vi "Auto_calibrate.vi"(3 "Mode":T4, 5 "Traverse line":T1 {"Carrier_2 Q (l/min)" format="%#.2f"; "Row Duration (mins)" format="%#.1f"; "Row No" min=0; "Trace Gas Concentration (%)" min=0.0 format="%#_4f"; "Carrier_1 Q (l/min)" format="%#.4f"; "Start X" format="%#.2f"; "Start Y" format="%#.2f"; "Start Z" format="%#.2f"; "End X" format="%#.2f"; "End Y" format="%#.2f"; "End Z" format="%#.2f"; "Tunnel Speed" format="%#.2f"; "Averaging time (mins)" min=0.0 format="%#.2f"}) -> (0 "Error Messages":string, 1 "Status":T6, 2 "Traverse Out":T1 {"Carrier_2 Q (l/min)" format="%#.2f"; "Row Duration (mins)" format="%#.1f"; "Row No" min=0; "Trace Gas Concentration (%)" min=0.0 format="%#_4f"; "Carrier_1 Q (l/min)" format="%#.4f"; "Start X" format="%#.2f"; "Start Y" format="%#.2f"; "Start Z" format="%#.2f"; "End X" format="%#.2f"; "End Y" format="%#.2f"; "End Z" format="%#.2f"; "Tunnel Speed" format="%#.2f"; "Averaging time (mins)" min=0.0 format="%#.2f"})   [LabVIEW 2022 SP3]
uses:
  Gen Trav/Traverse_cluster.ctl
  Gen Trav/Spacing.ctl
  Controls/Multi_run_mode.ctl
  Controls/User_Specific_mode.ctl
  Controls/Auto_Calib_Type.ctl
  Gen Trav/Multi_Run_Status.ctl
  Controls/Auto_Calib_Case.ctl
  FFID/HFR500 ppm Range.ctl
  File/Setup_Filetype.ctl
  Controls/Meas input Cluster.ctl
  Controls/Inst_type.ctl
  Controls/portOrDev.ctl
  Controls/calType.ctl
  Controls/channelState.ctl
  Controls/DAQinputType.ctl
  Controls/GMU Gas Line Name.ctl
  Gen Trav/Status_Cluster.ctl
  Calibration/Calib_mode.ctl
  ADAM Client/Sub VIs/ADAM Controls/Client_Source_Status.ctl
  Controls/Setup.ctl
  Controls/Post_Process.ctl
  Controls/Save_Data.ctl
  Controls/In_Range.ctl
  Controls/App_Global.ctl
  <vilib>/Analysis/baseanly.llb/Mean (DBL).vi
  Globals/Preference_global.vi
  Globals/Extra_Commands_Global.vi
  Globals/Meas_global.vi
  Globals/Calib_global.vi
  Globals/Trav_pos_global.vi
  Globals/Dynamic_call_global.ph.vi
  <vilib>/Analysis/NI_AALBase.lvlib
  <vilib>/Analysis/NI_AALPro.lvlib
panel:
  in  "stop":bool
  in  "Tab Control":enum32{"Page 1", "Page 2", "FFID"}(tab)
  out "Calibration varying":T5
  out "No of Calib Points":i32
  out "Currently On":i32
  out "Currently in Case":T7
  in  "Clear Calib History":bool
  out "New Calib Filenames":path[](array[path])
  out "Root Name":string[](array[string])
  out "Ch No's":string[](array[string])
  out "Wait factor":dbl
  out "Orig Calib file string":string
  out "Coefficients":dbl[][](array[numeric]) format="%.2f"
  out "Concentrations":dbl[](array[numeric])
  out "ppm/%Density":dbl[](array[numeric])
  out "FF Indexes":i16[](array[numeric])
  out "Values":dbl[][](array[numeric]) format="%.2f"
  out "FFID St Dev":dbl[][](array[numeric]) format="%.2f"
  out "Minimum St Dev":dbl[](array[numeric])
  out "Trace Gas %":dbl
  out "HFR500 Comms Channels":i32[](array[numeric])
  out "Multi FFID Range":bool
  in  "High Range ppm":T8=enum."5,000"
  in  "Slope less than":dbl=0.03
  in  "St Dev less than":dbl=0.25
  out "Calib Repeats":dbl[][][](array[numeric]) format="%#.3f"
  # "Specific Argument Options\n      Tunnel Speed;1;2;3;4\nOR  Traverse Position\nOR   Concentration"
  # "X           Y          Z"
  # "Start"
  # "End"
  # "X           Y          Z"
  # "Start"
  # "End"
  # "Value             St Dev        Slope Volts/min"
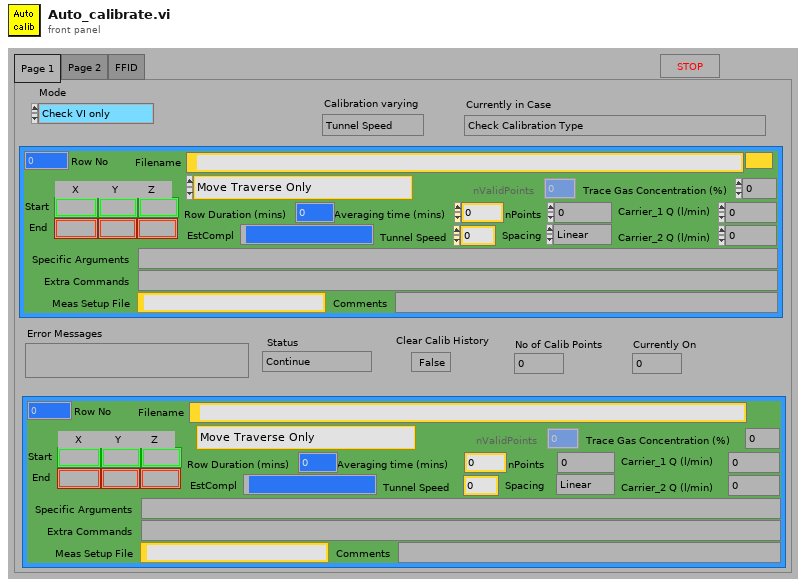
[diagram p1: front panel]
types:
  T1 = typedef "Traverse_cluster.ctl" = cluster{"Start X":sgl, "Start Y":sgl, "Start Z":sgl, "End X":sgl, "End Y":sgl, "End Z":sgl, "nPoints":i32, "Spacing":T2, "Filename":path, "Tunnel Speed":dbl, "Averaging time (mins)":dbl, "Extra Commands":string, "Carrier_1 Q (l/min)":dbl, "Carrier_2 Q (l/min)":dbl, "Trace Gas Concentration (%)":dbl, "Specific Arguments":string, "Comments":string, "Row No":i32, "Row Type Selector":T3, "EstCompl":string, "Row Duration (mins)":dbl, "nValidPoints":i32, "Meas Setup File":string}
  T2 = typedef "Spacing.ctl" = enum16{"Linear", "Log", "Gauss", "Specified", "N/A"}
  T3 = typedef "Multi_run_mode.ctl" = enum16{"Move Traverse Only", "Set Tunnel Speed Only", "Set Source Only", "Set Measurement Conditions", "Single Measurement", "Vertical Profile", "Lateral Profile", "Longitudinal Profile", "Multi-Axis Profile", "Explore Volume", "Auto Calibrate", "Meas Fast FID Bkgnd", "Check Beam Power", "Scanning Valve Measurement", "Run VI Named:", "Set ADAM Ch", "Wait (minutes)", "Send Message", "Synchronize With:", "Fall Back to this Row", "Turn Off Row Repeating", "Traverse 3D Volume", "Blank Row", "Jump to Fall Back Row"}
  T4 = typedef "User_Specific_mode.ctl" = enum16{"Check VI only", "Run VI"}
  T5 = typedef "Auto_Calib_Type.ctl" = enum16{"Tunnel Speed", "Traverse Position", "Concentration", "ESC RPM"}
  T6 = typedef "Multi_Run_Status.ctl" = enum16{"Continue", "Continue with Error", "Jump to Next Point", "Jump to Next Row", "Jump To Fall Back", "Terminate Run"}
  T7 = typedef "Auto_Calib_Case.ctl" = enum16{"Check Calibration Type", "Check if Original Calib file is Valid", "Get sampling rate etc. from meas setup file", "Setup Calibration Program", "Get Channel Numbers", "Check use latest selected on Mesurement setup files", "Create New Calib Filenames", "Setup Calibration Values in 2D array", "Create Measurement Setup File (Concentration Only)", "Are There Enough Calibration Points", "Set Measurement Conditions", "Measure Calibration Point", "Do Another Calibration Point?", "Skip Next Frame?", "Insert New calibration Filenames into Measurement Setup file", "Warn if FFID calibration is very non linear", "Warn if FFID voltages are too low", "Warn if FFID variance is high", "Insert Bkgnd Variance into calib file", "Warn if Current Calibration fit is poor", "Warn if Calibration Coefficients have significantly altered", "Reset Traverse positions", "Post Process Raw Data Files", "End"}
  T8 = typedef "HFR500 ppm Range.ctl" = enum16{"None", "1,000", "2,000", "5,000", "10,000", "20,000", "50,000", "100,000", "200,000"}
  T9 = typedef "Meas input Cluster.ctl" = cluster{"Type":T10, "Label":string, "DAQ":string, "Port":T11, "Ch":i32, "Cal":path, "calType":T12, "Fs":dbl, "syncDelay":dbl, "chState":T13, "inputConfig":T14}
  T10 = typedef "Inst_type.ctl" = enum16{"Raw voltage", "Raw with zero offsetting", "Propeller anemometer", "Pressure Transducer", "Pitot-static tube", "Hot wire", "Cross wire 1", "Cross wire 2", "Generic Linear", "Generic Polynomial", "Generic BackPoly", "Fast FID", "Thermocouple", "Cold wire", "Pulsed Wire", "LDA Vel", "LDA Tran time", "LDA Arr time", "Microphone"}
  T11 = typedef "portOrDev.ctl" = string
  T12 = typedef "calType.ctl" = enum32{"Latest", "Fixed"}
  T13 = typedef "channelState.ctl" = enum32{"No Selection", "Solo", "Mute"}
  T14 = typedef "DAQinputType.ctl" = string
  T15 = typedef "Setup_Filetype.ctl" = enum16{"Measurement Setups", "Calibration Setups", "General", "Results File Plotter Setups", "Speed Calib Tweaks"}
  T16 = typedef "GMU Gas Line Name.ctl" = enum16{"GMU1 Source", "GMU2 Source", "GMU2 Calib", "CPP GRC-A", "CPP GRC-B"}
  T17 = typedef "Status_Cluster.ctl" = cluster{"Status":T6, "Error Type":string, "Error Description":string}
  T18 = typedef "Calib_mode.ctl" = enum16{"Show Setup", "Take a New Calibration Point", "Refit Curve", "Setup Front Panel"}
  T19 = typedef "Client_Source_Status.ctl" = enum16{"Not Using", "Using", "Must Have"}
  T20 = typedef "Save_Data.ctl" = enum16{"Save No Data", "Save Data"}
  T21 = typedef "Post_Process.ctl" = enum16{"Take New Data", "Post Process Raw Data File"}
  T22 = typedef "Setup.ctl" = enum16{"Run Program", "Show Setup", "Save Current Setup", "Setup Front Panel"}
  T23 = typedef "In_Range.ctl" = enum16{"%", "±", "% & ±"}
  T24 = typedef "App_Global.ctl" = enum16{"Read Global", "Write to Global", "Initialise Array"}
  T25 = typedef "Cal_Inst_type.ctl" = enum16{"Propeller anemometer", "Pressure Transducer", "Hot wire", "Cross wire velocity", "Cross wire angle", "Generic Linear", "Generic Polynomial", "Poly Fit Special", "Fast FID", "Thermocouple", "Cold wire", "Pulsed Wire"}
  T26 = typedef "Ref_Inst_type.ctl" = enum16{"Propellor anemometer", "Pressure Transducer", "Raw voltage", "Pitot-static tube", "Generic Linear", "Generic Polynomial", "Thermocouple", "LDA", "Enter Value", "ADAM Channel"}
  T27 = cluster{"2nd Ref type":T26, "2nd inst present":bool}
  T28 = typedef "Calib Channel Setup.ctl" = cluster{"Ch No":i16, "Var name":string, "Device":string, "Port":string}
  T29 = typedef "Time_Trace_Cluster.ctl" = cluster{"Weighting":dbl[], "Voltage":dbl[], "Eng Values":dbl[]}
  T30 = typedef "Analysis_info_cluster.ctl" = cluster{"Colour":u32, "Inst type":T10, "Inst name":string, "Symbol":string, "Code name":string, "Extra Info":string, "Inst Array":T31, "U":dbl, "u^2":dbl, "u^3":dbl, "u^4":dbl, "Skew_u":dbl, "Kurt_u":dbl, "Sd Error in Mean":dbl, "% u'/U":dbl, "X":dbl, "Y":dbl, "Z":dbl, "Timescale integral Estimate":dbl, "Sd Error in Variance":dbl, "Calib File":path, "Calib Constants":dbl[], "Output Position":bool, "Stats":enum16{"None", "Basic", "Full"}, "Av Sampling Rate":dbl, "Av No of Samples":dbl, "Total Meas Time (s)":dbl, "OrigChName":string, "Max value":dbl, "Min value":dbl, "Req Sample Rate Hz":dbl, "Sync Delay Time (s)":dbl, "Ch No":i16, "Device":string, "Use Latest Calib":bool, "Port":string, "Metadata Ch Names":string[], "Metadata Ch Values":string[], "Label":string, "chState":T13, "Point Drift":dbl, "inputConfig":string}
  T31 = typedef "Instrument_Array.ctl" = enum16{"PWA", "LDA", "Analogue"}
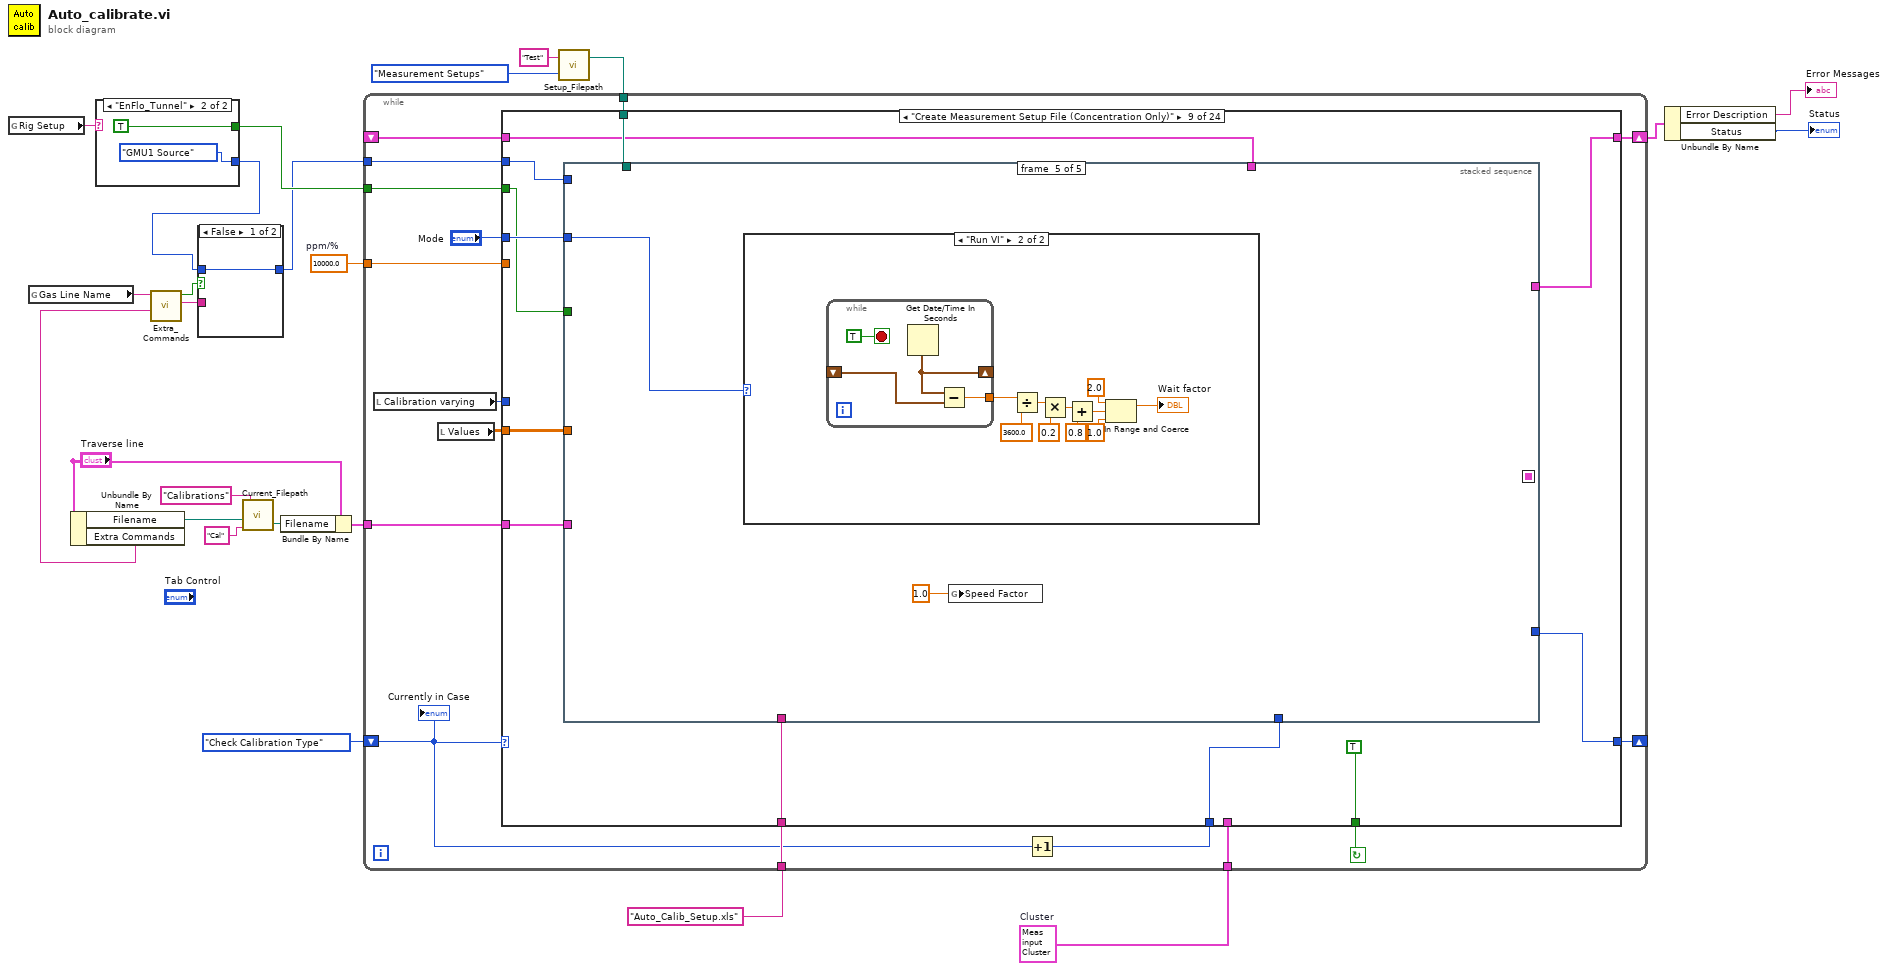
[diagram p0: block diagram]
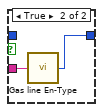
[diagram p2: hidden frame]
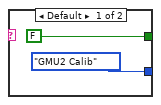
[diagram p3: hidden frame]
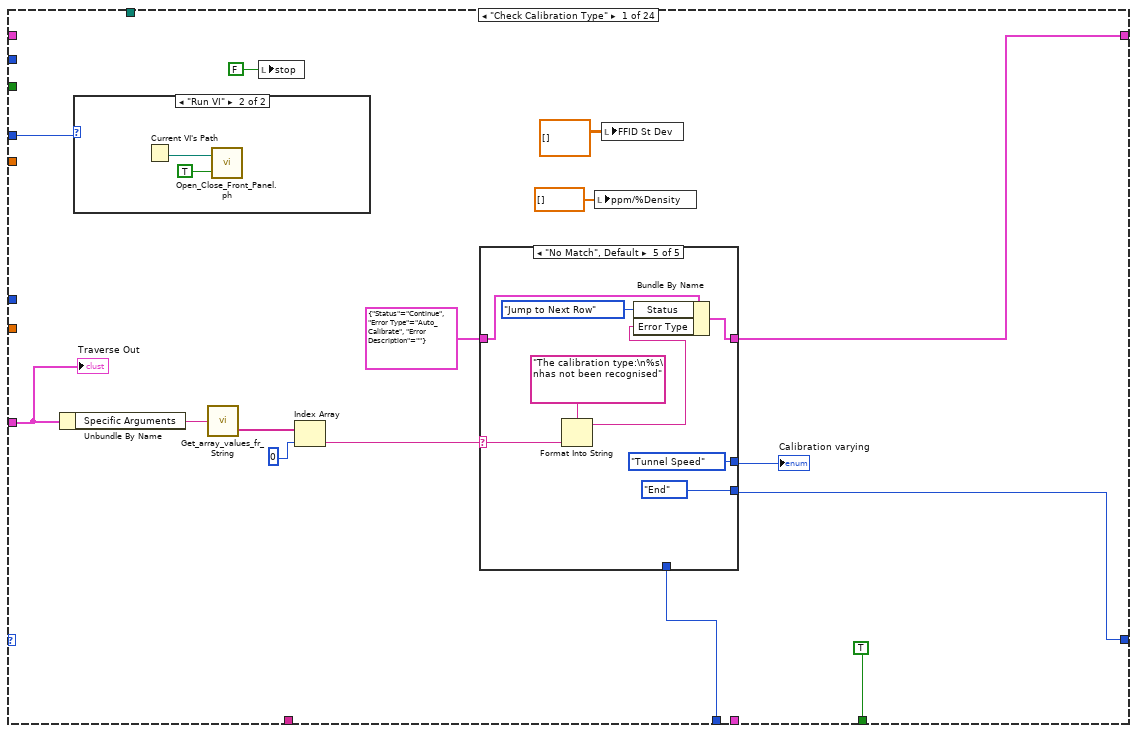
[diagram p4: hidden frame]
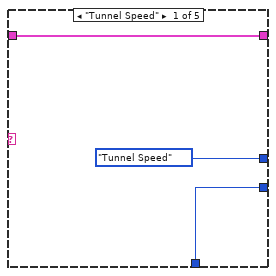
[diagram p6: hidden frame]
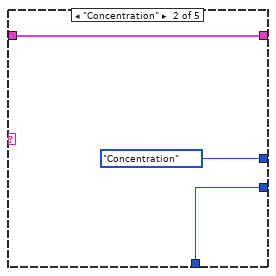
[diagram p7: hidden frame]
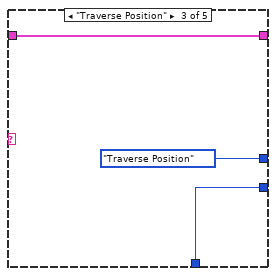
[diagram p8: hidden frame]
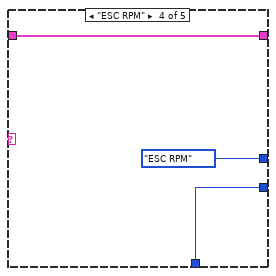
[diagram p9: hidden frame]
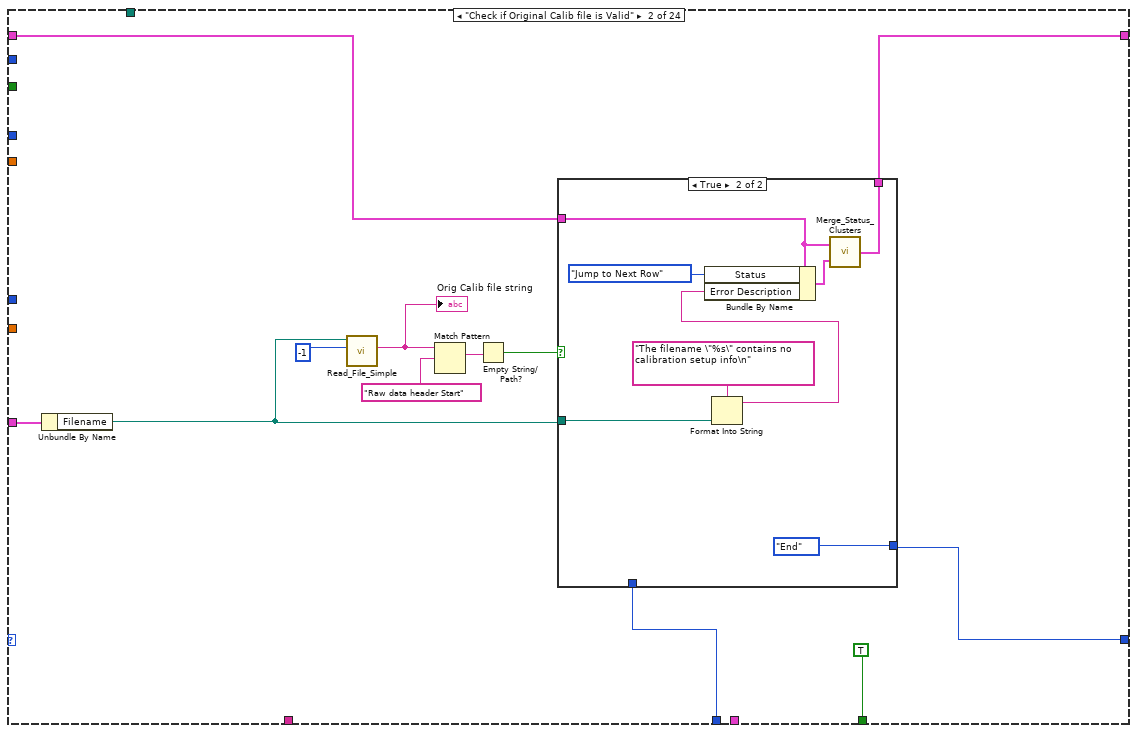
[diagram p10: hidden frame]
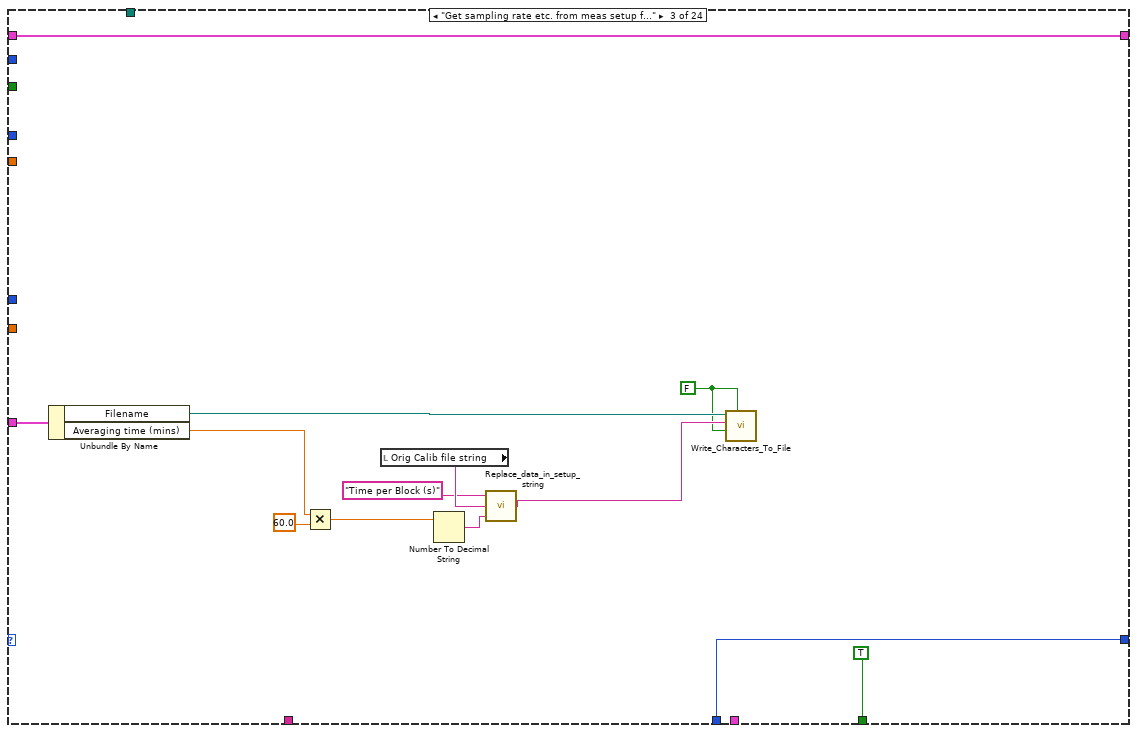
[diagram p12: hidden frame]
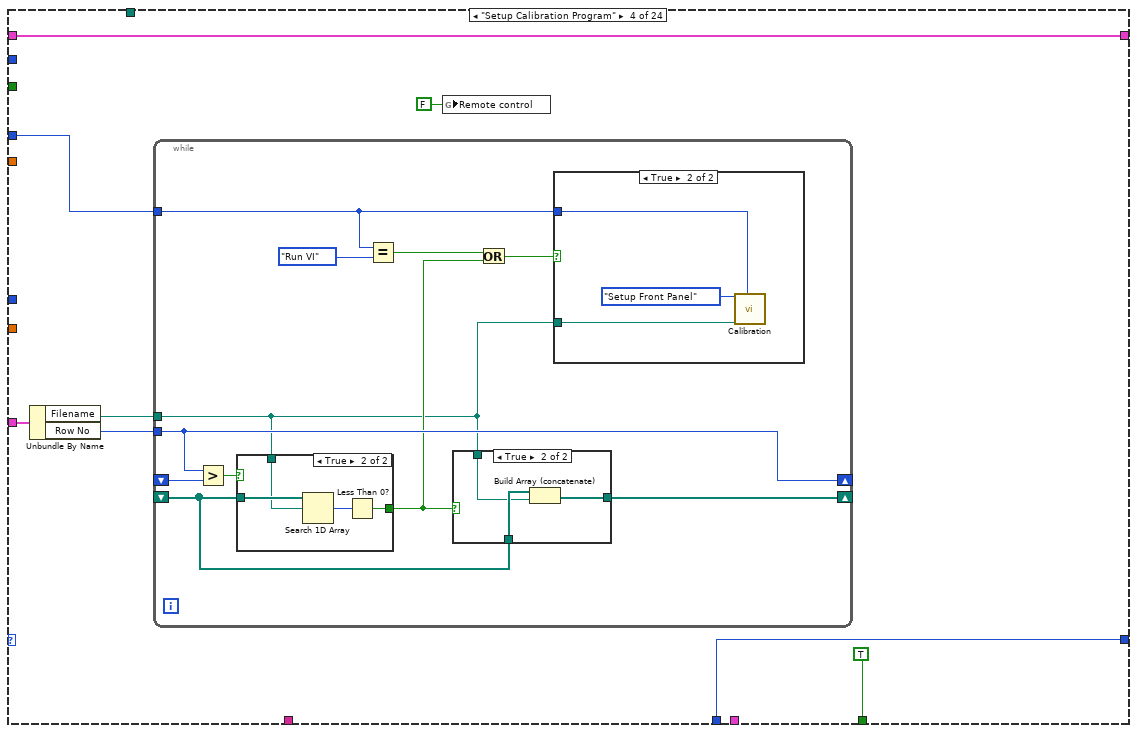
[diagram p13: hidden frame]
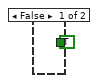
[diagram p16: hidden frame]
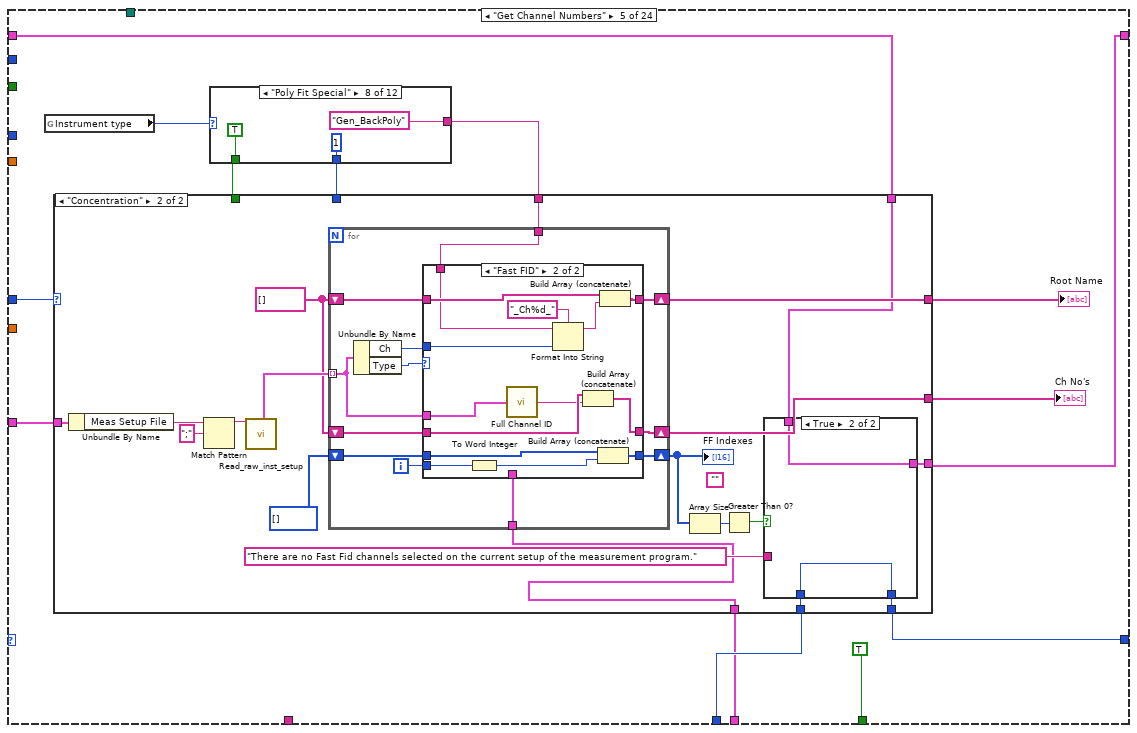
[diagram p17: hidden frame]
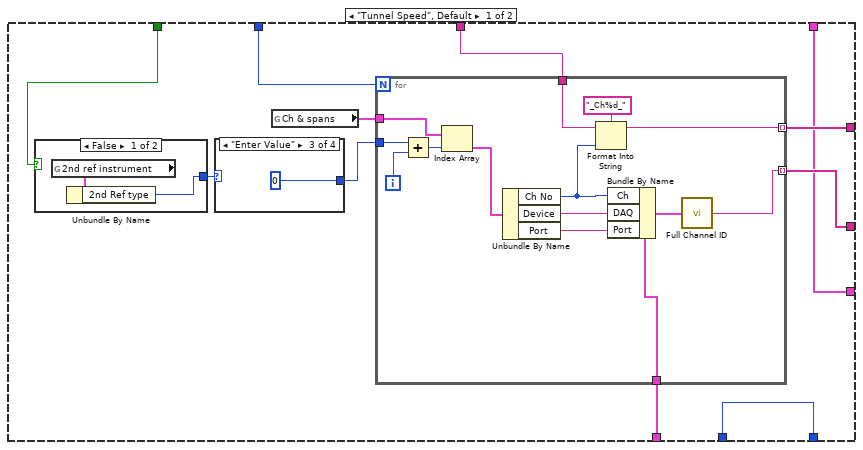
[diagram p18: hidden frame]
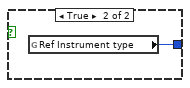
[diagram p19: hidden frame]
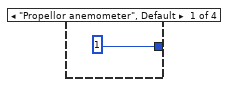
[diagram p20: hidden frame]
diagram:
  w1 = T9 {"Type"=enum."Raw voltage", "Label"="", "DAQ"="", "Port"="", "Ch"=0, "Cal"=path "", "calType"=enum."Latest", "Fs"=0.0, "syncDelay"=0.0, "chState"=enum."No Selection", "inputConfig"=""}  # Cluster
  w13 = 10000.0  # ppm/%
  n1 = global read "Preference_global.vi" "Rig Setup"() -> (w9:string)
  n2 = global read "Extra_Commands_Global.vi" "Gas Line Name"() -> (w7:string)
  n3 = Unbundle By Name("Traverse line") -> ("Filename"=w18:path, "Extra Commands"=w2:string)
  n4 = case shown="\"EnFlo_Tunnel\"" w9 {
    tunnel: [FALSE TRUE] -> w8
    tunnel: [GMU_Gas_Line_Name."GMU2 Calib" ("Gas Line Name") GMU_Gas_Line_Name."GMU1 Source" ("Gas Line Name")] -> w4
    frame Default {
    }
    frame "EnFlo_Tunnel" {
    }
  }
  n5 = call "Extra_Commands.vi"("String to Search"=w2, "Command"=w7) -> ("String Value"=w5:string, "Command Found"=w6:bool)  [unwired: 1 in, 3 out]
  n6 = case shown="False" w6 {
    tunnel: [w29 w30] -> w3
    tunnel: w5 -> [_ w31]
    tunnel: w4 -> [w29 _]
    frame False {
    }
    frame True {
      n7 = call "Gas line En-Type.vi"("Gas Line Name String"=w31) -> ("Gas Line Name"=w30:T16)  [unwired: 4 in]
    }
  }
  n8 = call "Current_Filepath.vi"("Short_Name"="Cal" ("Data Type"), "Filename in"=w18, "Data Type"="Calibrations") -> ("Filename Out"=w17:path)  [unwired: 1 in, 1 out]
  n9 = Bundle By Name(cluster="Traverse line", "Filename"=w17) -> (w15:T1)
  n10 = call "Setup_Filepath.vi"("Setup File Type"=Setup_Filetype."Measurement Setups", "Filename in"="Test") -> ("Directory"=w20:path)  [unwired: 1 out]
  n11 = while {
    shift-left: Auto_Calib_Case."Check Calibration Type" ("Currently in Case") -> [w41]
    shift-right: [w40] -> _
    tunnel: "Auto_Calib_Setup.xls" -> [w47]
    tunnel: w20 -> [w39]
    tunnel: w15 -> [w38]
    tunnel: w13 -> [w37]
    shift-right: [w36] -> w12
    shift-left: _ -> [w35]
    tunnel: w8 -> [w34]
    tunnel: w3 -> [w33]
    tunnel: w1 -> [w32]
    stop <- w44 continue-if-true
    n12 = local read "Calibration varying"() -> (w43:T5)
    n13 = local read "Values"() -> (w42:dbl[][])
    n14 = Increment(x=w41) -> (x+1=w45:T7)
    n15 = case shown="\"Create Measurement Setup File (Concentration Only)\"" w41 {
      tunnel: w38 -> [w50 w96 w119 w124 w158 _ w359 w415 w464 _ w624 w696 _ w1128 _ _ _ _ _ _ w1401 w1443 _ _]
      tunnel: "Mode" -> [w56 _ _ w125 _ _ w364 _ w465 _ w609 _ w1094 w1129 _ _ _ _ _ _ _ w1444 _ _]
      tunnel: w47 -> [_ _ _ _ _ _ _ _ w467 _ _ w707 _ _ _ _ _ _ _ _ _ _ _ _]
      tunnel: [w54 w89 w115 w127 w154 w298 w363 w404 w461 w592 w610 w706 w1095 w1132 w1160 w1175 w1236 w1280 w1339 w1359 w1423 w1447 w1480 w1483] -> w40
      tunnel: w45 -> [w55 w88 w115 w127 w153 w298 w363 w411 w460 w591 w611 w706 _ w1131 w1159 w1175 w1237 w1280 w1340 w1359 w1423 w1447 w1480 w1483]
      tunnel: [TRUE TRUE TRUE TRUE TRUE TRUE TRUE TRUE TRUE TRUE TRUE TRUE TRUE TRUE TRUE TRUE TRUE TRUE TRUE TRUE TRUE TRUE TRUE FALSE] -> w44
      tunnel: w43 -> [_ _ _ _ w161 _ w362 w413 _ _ w619 w708 _ w1130 w1155 _ _ _ _ _ _ w1445 _ _]
      tunnel: w42 -> [_ _ _ _ _ _ _ _ w463 w595 w623 w695 _ _ _ _ _ w1287 _ _ _ w1442 _ _]
      tunnel: w39 -> [_ _ _ _ _ w300 _ _ w466 _ _ _ _ _ _ _ _ _ _ _ _ _ _ _]
      tunnel: w37 -> [_ _ _ _ _ _ _ w409 _ _ _ w703 _ _ _ _ _ _ _ _ _ _ _ _]
      tunnel: [w49 w85 w107 w120 w155 w293 w356 w405 w459 w588 w613 w701 w1091 w1126 w1154 w1178 w1238 w1278 w1341 w1365 w1395 w1441 w1478 w1481] -> w36
      tunnel: w35 -> [_ w86 w107 w120 w156 w293 w356 w406 w458 w589 w615 w699 w1090 w1126 w1154 w1178 w1239 w1278 w1341 w1365 w1396 w1441 w1478 w1481]
      tunnel: w34 -> [_ _ _ _ _ _ _ _ w456 _ w606 w697 _ w1124 _ _ _ _ _ _ _ w1440 _ _]
      tunnel: w33 -> [_ _ _ _ _ _ _ _ w457 _ w608 w694 _ w1125 _ _ _ _ _ _ _ _ _ _]
      tunnel: w32 -> [_ _ _ _ w152 _ _ _ _ _ _ _ _ _ _ _ _ _ _ _ _ _ _ _]
      frame "Check Calibration Type" {
        n16 = Unbundle By Name(w50) -> ("Specific Arguments"=w62:string)
        n17 = case shown="\"Run VI\"" w56 {
          frame "Check VI only" {
          }
          frame "Run VI" {
            n18 = Current VI's Path() -> (path=w63:path)
            n19 = call "Open_Close_Front_Panel.ph.vi"("openWindow (T)"=TRUE ("Front Panel Window:Open"), "VI path"=w63) -> ()  [unwired: 1 in, 1 out]
          }
        }
        n20 = call "Get_array_values_fr_String.vi"("String Value"=w62) -> ("String array"=w61:string[])  [unwired: 1 out]
        n21 = local write "stop"(FALSE) -> ()
        n22 = Index Array(array=w61, index=0 ("Index")) -> (element=w59:string)
        n23 = case shown="\"No Match\", Default" w59 {
          selector: w59 -> [_ _ _ _ w81]
          tunnel: [Auto_Calib_Type."Tunnel Speed" ("Calibration varying") Auto_Calib_Type."Concentration" ("Calibration varying") Auto_Calib_Type."Traverse Position" ("Calibration varying") Auto_Calib_Type."ESC RPM" ("Calibration varying") Auto_Calib_Type."Tunnel Speed" ("Calibration varying")] -> w58
          tunnel: w55 -> [w66 w69 w72 w75 _]
          tunnel: [w66 w69 w72 w75 Auto_Calib_Case."End" ("Currently in Case")] -> w54
          tunnel: [w65 w68 w71 w74 w78] -> w49
          tunnel: T17 {"Status"=enum."Continue", "Error Type"="Auto_Calibrate", "Error Description"=""} ("Status Cluster 1") -> [w65 w68 w71 w74 w80]
          frame "Tunnel Speed" {
          }
          frame "Concentration" {
            (unwired) ""
          }
          frame "Traverse Position" {
          }
          frame "ESC RPM" {
          }
          frame "No Match", Default {
            n24 = Format Into String(format string="The calibration type:\n%s\nhas not been recognised" ("Format String"), w81) -> (resulting string=w79:string)  [unwired: 2 in, 1 out]
            n25 = Bundle By Name(cluster=w80, "Status"=Multi_Run_Status."Jump to Next Row", "Error Type"=w79) -> (w78:T17)
          }
        }
        "Calibration varying" <- w58
        n26 = local write "ppm/%Density"(dbl[] [] ("ppm/%Density")) -> ()
        n27 = local write "FFID St Dev"(dbl[][] [] ("FFID Variance")) -> ()
        "Traverse Out" <- w50
      }
      frame "Check if Original Calib file is Valid" {
        n28 = Unbundle By Name(w96) -> ("Filename"=w87:path)
        n29 = call "Read_File_Simple.vi"("Filename"=w87, "number of characters (all:-1)"=-1) -> ("string"=w93:string)  [unwired: 1 in, 7 out]
        "Orig Calib file string" <- w93
        n30 = Match Pattern(string=w93, regular expression="Raw data header Start") -> (match substring=w92:string)  [unwired: 4 out]
        n31 = Empty String/Path?(string/path=w92) -> (empty?=w91:bool)
        n32 = case shown="True" w91 {
          tunnel: w87 -> [_ w106]
          tunnel: [w98 Auto_Calib_Case."End" ("Currently in Case")] -> w89
          tunnel: w88 -> [w98 _]
          tunnel: w86 -> [w97 w103]
          tunnel: [w97 w99] -> w85
          frame False {
          }
          frame True {
            n33 = Format Into String(format string="The filename \"%s\" contains no calibration setup info\n" ("Format String"), w106) -> (resulting string=w100:string)  [unwired: 2 in, 1 out]
            n34 = Bundle By Name(cluster=w103, "Status"=Multi_Run_Status."Jump to Next Row", "Error Description"=w100) -> (w101:T17)
            n35 = call "Merge_Status_Clusters.vi"("Status Cluster 2"=w101, "Status Cluster 1"=w103) -> ("Status Cluster Out"=w99:T17)
          }
        }
      }
      frame "Get sampling rate etc. from meas setup file" {
        w108 = FALSE ("advisory dialog? (display:T)")
        n36 = Unbundle By Name(w119) -> ("Filename"=w117:path, "Averaging time (mins)"=w109:dbl)
        n37 = Multiply(x=w109, y=60.0 ("x")) -> (x*y=w113:dbl)
        n38 = local read "Orig Calib file string"() -> (w112:string)
        n39 = Number To Decimal String(number=w113) -> (decimal integer string=w110:string)  [unwired: 1 out]
        n40 = call "Replace_data_in_setup_string.vi"("New data string"=w110, "Input string"=w112, "Variable name"="Time per Block (s)") -> ("Appended string"=w116:string)
        n41 = call "Write_Characters_To_File.vi"("file path (dialog if empty)"=w117, "advisory dialog? (display:T)"=w108, "character string"=w116, "append to file? (new file:F)"=w108) -> ()  [unwired: 1 in, 4 out]
      }
      frame "Setup Calibration Program" {
        n42 = Unbundle By Name(w124) -> ("Filename"=w121:path, "Row No"=w123:i32)
        n43 = while {
          shift-left: _ -> [w131]
          shift-right: [w130] -> _
          tunnel: w123 -> [w138]
          shift-left: _ -> [w139]
          shift-right: [w138] -> _
          tunnel: w125 -> [w136]
          tunnel: w121 -> [w128]
          stop <- FALSE continue-if-true
          n44 = Greater?(x=w138, y=w139) -> (0:w137:bool)
          n45 = case shown="True" w137 {
            tunnel: w131 -> [_ w151]
            tunnel: w128 -> [_ w150]
            tunnel: [TRUE w148] -> w132
            frame False {
            }
            frame True {
              n46 = Search 1D Array(1D array=w151, element=w150) -> (index of element=w149:i32)  [unwired: 1 out]
              n47 = Less Than 0?(x=w149) -> (x < 0?=w148:bool)
            }
          }
          n48 = Equal?(x=w136, y=User_Specific_mode."Run VI" ("Mode")) -> (x = y?=w134:bool)
          n49 = case shown="True" w132 {
            tunnel: w131 -> [w140 w143]
            tunnel: w128 -> [_ w142]
            tunnel: [w140 w141] -> w130
            frame False {
            }
            frame True {
              n50 = Build Array (concatenate)(w143, w142) -> (w141:path[])
            }
          }
          n51 = Or(x=w134, y=w132) -> (x .or. y?=w133:bool)
          n52 = case shown="True" w133 {
            tunnel: w136 -> [_ w146]
            tunnel: w128 -> [_ w145]
            frame False {
            }
            frame True {
              n53 = call "Calibration.vi"("Mode"=Calib_mode."Setup Front Panel", "Calib file"=w145, "Simulate/Run"=w146) -> ()  [unwired: 17 out]
            }
          }
        }
        n54 = global write "Meas_global.vi" "Remote control"(FALSE ("Remote control")) -> ()
      }
      frame "Get Channel Numbers" {
        n55 = global read "Calib_global.vi" "Instrument type"() -> (w165:T25)
        n56 = case shown="\"Poly Fit Special\"" w165 {
          tunnel: ["Prop" "Mano" "HW" "XW" "XW" "Gen_Lin" "Gen_Poly" "Gen_BackPoly" "FF" "Therm" "CW" "PWA"] -> w164
          tunnel: [1 1 1 2 2 1 1 1 1 1 1 1] -> w159
          tunnel: [TRUE TRUE TRUE TRUE FALSE TRUE TRUE TRUE TRUE TRUE TRUE TRUE] -> w157
          frame "Propeller anemometer" {
          }
          frame "Pressure Transducer" {
          }
          frame "Hot wire" {
          }
          frame "Cross wire velocity" {
          }
          frame "Cross wire angle" {
          }
          frame "Generic Linear" {
          }
          frame "Generic Polynomial" {
          }
          frame "Poly Fit Special" {
          }
          frame "Fast FID" {
          }
          frame "Thermocouple" {
          }
          frame "Cold wire" {
          }
          frame "Pulsed Wire" {
          }
        }
        n57 = case shown="\"Concentration\"" w161 {
          tunnel: w164 -> [w175 w216]
          tunnel: [w171 w215] -> w163
          tunnel: [w172 w214] -> w162
          tunnel: w159 -> [w173 _]
          tunnel: w158 -> [_ w210]
          tunnel: w157 -> [w169 _]
          tunnel: w156 -> [w168 w203]
          tunnel: [w168 w202] -> w155
          tunnel: [w167 w201] -> w154
          tunnel: w153 -> [w167 w200]
          tunnel: w152 -> [w166 w199]
          frame "Tunnel Speed", Default {
            n58 = case shown="False" w169 {
              tunnel: [w177 w179] -> w176
              frame False {
                n59 = global read "Calib_global.vi" "2nd ref instrument"() -> (w178:T27)
                n60 = Unbundle By Name(w178) -> ("2nd Ref type"=w177:T26)
              }
              frame True {
                n61 = global read "Calib_global.vi" "Ref Instrument type"() -> (w179:T26)
              }
            }
            n62 = case shown="\"Enter Value\"" w176 {
              tunnel: [1 0 0 0] -> w170
              frame "Propellor anemometer", Default {
              }
              frame "LDA" {
              }
              frame "Enter Value" {
              }
              frame "ADAM Channel" {
              }
            }
            n63 = global read "Calib_global.vi" "Ch & spans"() -> (w174:T28[])
            n64 = for {
              N: w173 -> [_]
              tunnel: [w181] -> w172 mode=indexing
              tunnel: w175 -> [w191]
              tunnel: w174 -> [w190]
              tunnel: [w189] -> w171 mode=indexing
              tunnel: w170 -> [w187]
              tunnel: w166 -> [w180]
              i -> [w188]
              n65 = Add(x=w187, y=w188) -> (x+y=w186:i32)
              n66 = Index Array(array=w190, index=w186) -> (element=w193:T28)
              n67 = Unbundle By Name(w193) -> ("Ch No"=w184:i16, "Device"=w183:string, "Port"=w182:string)
              n68 = Format Into String(format string="_Ch%d_" ("Format String"), initial string=w191, w184) -> (resulting string=w189:string)  [unwired: 1 in, 1 out]
              n69 = Bundle By Name(cluster=w180, "Ch"=w184, "DAQ"=w183, "Port"=w182) -> (w185:T9)
              n70 = call "Full Channel ID.vi"("Cluster"=w185) -> ("String"=w181:string)
            }
          }
          frame "Concentration" {
            (unwired) ""
            w198 = string[] []
            n71 = Unbundle By Name(w210) -> ("Meas Setup File"=w207:string)
            n72 = Match Pattern(string=w207, regular expression=";") -> (before substring=w206:string)  [unwired: 4 out]
            n73 = call "Read_raw_inst_setup.vi"("Setup file"=w206) -> ("Ch & spans choices"=w209:T9[])  [unwired: 18 out]
            n74 = for {
              tunnel: w209 -> [w225] mode=indexing
              tunnel: w216 -> [w236]
              shift-right: [w232] -> w215
              shift-left: w198 -> [w233]
              shift-right: [w230] -> w214
              shift-left: w198 -> [w231]
              shift-right: [w229] -> w212
              shift-left: i16[] [] -> [w228]
              tunnel: w199 -> [w226]
              i -> [w227]
              n75 = Unbundle By Name(w225) -> ("Ch"=w235:i32, "Type"=w234:T10)
              n76 = case shown="\"Fast FID\"" w234 {
                tunnel: w236 -> [_ w244]
                tunnel: w235 -> [_ w242]
                tunnel: w233 -> [w239 w253]
                tunnel: [w239 w252] -> w232
                tunnel: w231 -> [w238 w251]
                tunnel: [w238 w250] -> w230
                tunnel: w228 -> [w237 w248]
                tunnel: [w237 w249] -> w229
                tunnel: w227 -> [_ w247]
                tunnel: w226 -> [_ _]
                tunnel: w225 -> [_ w240]
                frame "Generic Linear", Default {
                }
                frame "Fast FID" {
                  n77 = To Word Integer(number=w247) -> (16bit integer=w246:i16)
                  n78 = call "Full Channel ID.vi"("Cluster"=w240) -> ("String"=w241:string)
                  n79 = Format Into String(format string="_Ch%d_", initial string=w244, w242) -> (resulting string=w243:string)  [unwired: 1 in, 1 out]
                  n80 = Build Array (concatenate)(w251, w241) -> (w250:string[])
                  n81 = Build Array (concatenate)(w248, w246) -> (w249:i16[])
                  n82 = Build Array (concatenate)(w253, w243) -> (w252:string[])
                }
              }
            }
            "FF Indexes" <- w212
            n83 = Array Size(array=w212) -> (size(s)=w211:i32)
            n84 = Greater Than 0?(x=w211) -> (x > 0?=w205:bool)
            n85 = case shown="True" w205 {
              tunnel: "There are no Fast Fid channels selected on the current setup of the measurement program." ("f") -> [w221 _]
              tunnel: w203 -> [w219 w224]
              tunnel: [w218 w224] -> w202
              tunnel: [Auto_Calib_Case."End" ("Currently in Case") w223] -> w201
              tunnel: w200 -> [_ w223]
              frame False {
                n86 = Bundle By Name(cluster=w219, "Status"=Multi_Run_Status."Jump to Next Row", "Error Description"=w221) -> (w220:T17)
                n87 = call "Merge_Status_Clusters.vi"("Status Cluster 2"=w220, "Status Cluster 1"=w219) -> ("Status Cluster Out"=w218:T17)
              }
              frame True {
              }
            }
          }
        }
        "Root Name" <- w163
        "Ch No's" <- w162
      }
      frame "Check use latest selected on Mesurement setup files" {
        n88 = global read "Trav_pos_global.vi" "Measurement setup files"() -> (w294:string[])
        n89 = local read "Ch No's"() -> (w299:string[])
        n90 = Build Array (concatenate)(w294, "Current_Setup.xls") -> (w295:string[])
        n91 = for {
          tunnel: w300 -> [w308]
          tunnel: w295 -> [w307] mode=indexing
          tunnel: w299 -> [w306]
          shift-right: [w304] -> w290
          shift-left: "" -> [w305]
          n92 = stacked-sequence {
            seq-local: [w310 _ _] -> [_ w320 _]
            seq-local: [w309 _ _] -> [_ w319 _]
            seq-local: [_ w317 _] -> [_ _ w345]
            tunnel: w308 -> [w314 _ _]
            tunnel: w307 -> [w313 _ w346]
            tunnel: w306 -> [_ w321 _]
            tunnel: w305 -> [_ _ w344]
            tunnel: [_ _ w343] -> w304
            frame #0 {
              n93 = Build Path(base path=w314, name or relative path=w313) -> (appended path=w312:path)
              n94 = Read from Text File(file (use dialog)=w312) -> (text=w311:string)  [unwired: 3 in, 3 out]
              n95 = call "Analysis Info Cluster from String.vi"("Setup String"=w311) -> ("Ch & spans choices"=w309:T9[])  [unwired: 7 out]
              n96 = for {
                tunnel: w309 -> [w315] mode=indexing
                tunnel: [w316] -> w310 mode=indexing
                n97 = call "Full Channel ID.vi"("Cluster"=w315) -> ("String"=w316:string)
              }
            }
            frame #1 {
              n98 = for {
                tunnel: w321 -> [w324] mode=indexing
                tunnel: w320 -> [w328]
                tunnel: w319 -> [w327]
                shift-right: [w322] -> w317
                shift-left: "" -> [w323]
                n99 = Search 1D Array(1D array=w328, element=w324) -> (index of element=w325:i32)  [unwired: 1 in]
                n100 = Greater Or Equal To 0?(x=w325) -> (x >= 0?=w326:bool)
                n101 = case shown="True" w326 {
                  tunnel: w327 -> [_ w337]
                  tunnel: w325 -> [_ w336]
                  tunnel: w324 -> [_ w333]
                  tunnel: w323 -> [w329 w332]
                  tunnel: [w329 w331] -> w322
                  frame False {
                  }
                  frame True {
                    n102 = Index Array(array=w337, index=w336) -> (element=w335:T9)
                    n103 = Unbundle By Name(w335) -> ("calType"=w334:T12)
                    n104 = case shown="\"Fixed\"" w334 {
                      tunnel: w333 -> [_ w341]
                      tunnel: w332 -> [w338 w342]
                      tunnel: [w338 w340] -> w331
                      tunnel: " is not set to use the latest Calibration " -> [_ w339]
                      frame "Latest" {
                      }
                      frame "Fixed" {
                        n105 = Concatenate Strings(w342, w341, w339) -> (w340:string)
                      }
                    }
                  }
                }
              }
            }
            frame #2 {
              n106 = Empty String/Path?(string/path=w345) -> (empty?=w347:bool)
              n107 = case shown="True" w347 {
                tunnel: w346 -> [w353 _]
                tunnel: w345 -> [w351 _]
                tunnel: w344 -> [w350 w354]
                tunnel: [w348 w354] -> w343
                frame False {
                  n108 = Format Into String(format string="in Measurement Setup File %s.\n", initial string=w351, w353) -> (resulting string=w349:string)  [unwired: 1 in, 1 out]
                  n109 = Concatenate Strings(w350, w349) -> (w348:string)
                }
                frame True {
                }
              }
            }
          }
        }
        n110 = Empty String/Path?(string/path=w290) -> (empty?=w291:bool)
        n111 = case shown="False" w291 {
          tunnel: w290 -> [w301 _]
          frame False {
            w303 = errorcluster {"status"=FALSE, "code"=0, "source"=""} ("error in (no error)")
            n112 = Bundle By Name(cluster=w303, "status"=TRUE, "source"=w301) -> ()  [unwired: 1 out]
            n113 = call "EnFlo_Error_Handler.vi"("error in (no error)"=w303) -> ()  [unwired: 2 in, 3 out]
          }
          frame True {
          }
        }
      }
      frame "Create New Calib Filenames" {
        n114 = Unbundle By Name(w359) -> ("Filename"=w358:path)
        n115 = local read "Root Name"() -> (w361:string[])
        n116 = case shown="\"Concentration\"" w362 {
          tunnel: w361 -> [_ w376]
          tunnel: [1 w375] -> w360
          frame "Tunnel Speed", Default {
          }
          frame "Concentration" {
            n117 = Array Size(array=w376) -> (size(s)=w375:i32)
          }
        }
        n118 = Strip Path(path=w358) -> (stripped path=w357:path)  [unwired: 1 out]
        n119 = Get Date/Time String(date format (0)=enum16{"short", "long", "abbreviated"}."short") -> (date string=w368:string)  [unwired: 3 out]
        n120 = call "getFileExtPreference.vi"() -> ("Suffix to add"=w355:string)  [unwired: 11 in]
        n121 = call "Replace_Character.vi"("Replace with"="-", "Input String"=w368, "Search For"="/") -> ("Output string"=w365:string)  [unwired: 1 out]
        n122 = for {
          N: w360 -> [_]
          tunnel: w361 -> [w381] mode=indexing
          tunnel: w357 -> [w378]
          tunnel: [w380] -> w372 mode=indexing
          tunnel: w365 -> [w382]
          tunnel: w364 -> [w379]
          tunnel: w355 -> [w377]
          n123 = while {
            tunnel: w381 -> [w394]
            tunnel: w382 -> [w395]
            tunnel: [w390] -> w383
            tunnel: w378 -> [w388]
            tunnel: w377 -> [w386]
            i -> [w398]
            stop <- w400 continue-if-true
            n124 = Increment(x=w398) -> (x+1=w396:i32)
            n125 = Format Into String(format string="%s_%d%s" ("Format String"), initial string=w394, w395, w396, w386) -> (resulting string=w391:string)  [unwired: 1 in, 1 out]
            n126 = List Folder(path=w388) -> (filenames=w389:string[])  [unwired: 1 in, 5 out]
            n127 = call "Replace_Character.vi"("Replace with"="_", "Input String"=w391, "Search For"=" ") -> ("Output string"=w390:string)  [unwired: 1 out]
            n128 = To Upper Case(1:w389) -> (0:w387:string[])
            n129 = To Upper Case(1:w390) -> (0:w399:string)
            n130 = Search 1D Array(1D array=w387, element=w399) -> (index of element=w401:i32)  [unwired: 1 out]
            n131 = Not Equal?(x=w401, y=-1) -> (x != y?=w400:bool)
          }
          n132 = Build Path(base path=w378, name or relative path=w383) -> (appended path=w380:path)
          n133 = case shown="\"Run VI\"" w379 {
            tunnel: w380 -> [_ w384]
            frame "Check VI only" {
            }
            frame "Run VI" {
              n134 = call "Calibration.vi"("Mode"=Calib_mode."Setup Front Panel", "Calib file"=w384) -> ()  [unwired: 1 in, 17 out]
            }
          }
        }
        "New Calib Filenames" <- w372
        n135 = Index Array(array=w372, index=0 ("Index")) -> (element=w370:path)
        n136 = global write "Meas_global.vi" "Results file"(w370) -> ()
      }
      frame "Setup Calibration Values in 2D array" {
        n137 = case shown="\"Tunnel Speed\", \"ESC RPM\"" w413 {
          tunnel: [w433 w444 w455] -> w412
          tunnel: w415 -> [w428 w442 w454]
          tunnel: ["" w436 w453] -> w407
          tunnel: w411 -> [w427 w445 w452]
          tunnel: [w426 w445 w451] -> w403
          tunnel: [dbl[] [] w443 dbl[] []] -> w410
          tunnel: w409 -> [_ w437 _]
          frame "Tunnel Speed", "ESC RPM" {
            n138 = Unbundle By Name(w428) -> ("Specific Arguments"=w431:string)
            n139 = call "Get_array_values_fr_String.vi"("String Value"=w431) -> ("Numeric Array"=w429:dbl[])  [unwired: 1 out]
            n140 = Array Subset(array=w429, index=1 ("Array Index")) -> (w425:dbl[])  [unwired: 1 in]
            n141 = for {
              tunnel: w425 -> [w435] mode=indexing
              tunnel: [w434] -> w433 mode=indexing
              n142 = Build Array(w435) -> (w434:dbl[])
            }
            n143 = Increment(x=w427) -> (x+1=w426:T7)
          }
          frame "Concentration" {
            n144 = Unbundle By Name(w442) -> ("Specific Arguments"=w441:string)
            n145 = call "Read_FFID_Auto_Calib_Setup.vi"("Specific Argument"=w441) -> ("Trace concentration %"=w438:dbl[], "Carrier 2 Q"=w439:dbl[], "Carrier 1 Q"=w440:dbl[], "Error String"=w436:string)  [unwired: 1 out]
            n146 = for {
              tunnel: w440 -> [w449] mode=indexing
              tunnel: [w448] -> w444 mode=indexing
              tunnel: w439 -> [w447] mode=indexing
              tunnel: w438 -> [w446] mode=indexing
              n147 = Build Array(w449, w447, w446) -> (w448:dbl[])
            }
            n148 = Multiply(x=w437, y=w438) -> (x*y=w443:dbl[])
          }
          frame "Traverse Position" {
            n149 = call "Create_Pos_array.vi"("Traverse line"=w454) -> ("Error Messages"=w453:string, "Array of Positions"=w455:sgl[][])  [unwired: 5 in, 2 out]
            n150 = Increment(x=w452) -> (x+1=w451:T7)
          }
        }
        "Values" <- w412
        "Concentrations" <- w410
        n151 = Empty String/Path?(string/path=w407) -> (empty?=w408:bool)
        n152 = case shown="True" w408 {
          tunnel: w407 -> [w421 _]
          tunnel: w406 -> [w419 w423]
          tunnel: [w417 w423] -> w405
          tunnel: [Auto_Calib_Case."End" ("Currently in Case") w422] -> w404
          tunnel: w403 -> [_ w422]
          frame False {
            n153 = Bundle By Name(cluster=w419, "Error Description"=w421, "Status"=Multi_Run_Status."Jump to Next Row") -> (w418:T17)
            n154 = call "Merge_Status_Clusters.vi"("Status Cluster 2"=w418, "Status Cluster 1"=w419) -> ("Status Cluster Out"=w417:T17)
          }
          frame True {
          }
        }
      }
      frame "Create Measurement Setup File (Concentration Only)" {
        n155 = stacked-sequence {
          seq-local: [_ _ w503 _ _] -> [_ _ _ w527 _]
          tunnel: w466 -> [_ _ _ _ _]
          tunnel: w467 -> [_ w479 _ _ _]
          tunnel: w465 -> [w468 _ w505 w526 w573]
          tunnel: w464 -> [_ w472 w504 _ _]
          tunnel: w463 -> [_ _ w506 _ _]
          tunnel: [_ _ _ w525 _] -> w461
          tunnel: w460 -> [_ _ _ w524 _]
          tunnel: w458 -> [_ _ _ w523 _]
          tunnel: [_ _ _ w522 _] -> w459
          tunnel: w457 -> [_ _ _ w520 _]
          tunnel: w456 -> [_ _ w502 w519 _]
          frame #0 {
            n156 = case shown="\"Check VI only\"" w468 {
              frame "Check VI only" {
              }
              frame "Run VI" {
                w469 = u32 1  # Time to hold source OFF (microseconds)
                w470 = u32 0  # Time to hold source ON (microseconds)
                n157 = call "Arduino_Timed_Release.vi"("Time to hold source ON (microseconds)"=w470, "Time to hold source OFF (microseconds)"=w469, "Number of cycles"=u16 1) -> ()  [unwired: 2 out]
              }
            }
          }
          frame #1 {
            n158 = global read "Meas_global.vi" "Results file"() -> (w474:path)
            n159 = Strip Path(path=w474) -> (name=w473:string)  [unwired: 1 out]
            n160 = call "Create FFID Auto Calib setup file.vi"("Results filename"=w473, "Auto_Calib_Setup.xls"=w479, "Traverse line"=w472) -> ("HFR500 Comms Channels"=w478:string[])  [unwired: 3 in]
            n161 = for {
              tunnel: w478 -> [w501] mode=indexing
              tunnel: [w500] -> w477 mode=indexing
              tunnel: [w499] -> w475 mode=indexing
              n162 = Decimal String To Number(string=w501) -> (number=w500:i32)  [unwired: 2 in, 1 out]
              n163 = Greater Than 0?(x=w500) -> (x > 0?=w499:bool)
            }
            "HFR500 Comms Channels" <- w477
            n164 = Or Array Elements(Boolean array=w475) -> (logical OR=w476:bool)
            "Multi FFID Range" <- w476
            n165 = case shown="True" w476 {
              tunnel: w475 -> [_ w483]
              frame False {
              }
              frame True {
                n166 = local read "New Calib Filenames"() -> (w482:path[])
                n167 = for {
                  tunnel: w483 -> [w484] mode=indexing
                  tunnel: w482 -> [w486] mode=indexing
                  tunnel: [w485] -> w481 mode=indexing if=w484
                  n168 = case shown="True" w484 {
                    tunnel: w486 -> [w487 w498]
                    tunnel: [w487 w488] -> w485
                    frame False {
                    }
                    frame True {
                      n169 = Strip Path(path=w498) -> (stripped path=w489:path, name=w494:string)
                      n170 = String Length(string=w494) -> (length=w496:i32)
                      n171 = Subtract(x=w496, y=4 ("offset (0)")) -> (x-y=w495:i32)
                      n172 = Search/Split String(string=w494, offset (0)=w495) -> (substring before match=w492:string, match + rest of string=w493:string)  [unwired: 1 in, 1 out]
                      n173 = Concatenate Strings(w492, "H" ("string"), w493) -> (w490:string)
                      n174 = Build Path(base path=w489, name or relative path=w490) -> (appended path=w488:path)
                    }
                  }
                }
                n175 = Build Array (concatenate)(w482, w481) -> (w480:path[])
                n176 = local write "New Calib Filenames"(w480) -> ()
              }
            }
          }
          frame #2 {
            n177 = case shown="\"Run VI\"" w505 {
              tunnel: w506 -> [w515 _]
              tunnel: w504 -> [w514 w518]
              tunnel: [w513 w518] -> w503
              tunnel: w502 -> [w512 _]
              frame "Run VI" {
                (unwired) "GMU:Mains Divertor:Valve"
                # "#SiteSpecific -Will need generalising..."
                n178 = case shown="True" w512 {
                  frame False {
                  }
                  frame True {
                    n179 = call "ASYNC_Adam_client.vi"("Values"=dbl[] [1.0], "Channel Names"=string[] ["GMU:Mains Divertor:Valve"]) -> ()  [unwired: 1 in, 2 out]
                  }
                }
                n180 = Index Array(array=w515, index (row)=0) -> (element=w510:dbl[])  [unwired: 1 in]
                n181 = Index Array(array=w510) -> (element #1=w508:dbl, element #2=w509:dbl, element #3=w507:dbl)  [unwired: 3 in]
                n182 = Bundle By Name(cluster=w514, "Carrier_1 Q (l/min)"=w508, "Carrier_2 Q (l/min)"=w509, "Trace Gas Concentration (%)"=w507) -> (w513:T1)
              }
              frame "Check VI only" {
              }
            }
          }
          frame #3 {
            w529 = dbl[] [0.0, 0.0, 0.0, 0.0]  # X Offset
            w531 = dbl[] [60.0, 30.0, 15.0, 0.0]  # Z Offset
            n183 = Unbundle By Name(w527) -> ("Start X"=w528:sgl, "Start Z"=w530:sgl)
            n184 = stacked-sequence {
              tunnel: w527 -> [w536 _]
              tunnel: w526 -> [w535 _]
              tunnel: w520 -> [w534 _]
              tunnel: w519 -> [_ w537]
              frame #0 {
                n185 = call "Set_Source.vi"("Source Establishment Time (s)"=15.0, "Source Status"=Client_Source_Status."Using", "Gas Line Name"=w534, "Traverse line"=w536, "Simulate/Run"=w535) -> ()  [unwired: 6 out]
              }
              frame #1 {
                n186 = case shown="True" w537 {
                  frame False {
                  }
                  frame True {
                    n187 = call "ASYNC_Adam_client.vi"("Values"=dbl[] [3.0], "Channel Names"=string[] ["Clean_Air:Hi-Tec:Dem Volt"]) -> ()  [unwired: 1 in, 2 out]
                  }
                }
              }
            }
            n188 = for {
              tunnel: w526 -> [w546]
              tunnel: w527 -> [w559]
              tunnel: w531 -> [w558] mode=indexing
              tunnel: w530 -> [w556]
              tunnel: w529 -> [w555] mode=indexing
              tunnel: w528 -> [w554]
              tunnel: [w541] -> w525
              tunnel: w524 -> [w540]
              tunnel: [w542] -> w521
              i -> [w551]
              stop <- w543 continue-if-true
              n189 = Greater?(x=w551, y=1) -> (0:w550:bool)
              n190 = case shown="True" w550 {
                tunnel: ["No Backlash" ""] -> w549
                tunnel: [1.0 ("f") 0.5 ("t")] -> w548
                frame False {
                }
                frame True {
                }
              }
              n191 = Add(x=w554, y=w555) -> (x+y=w553:dbl)
              n192 = Add(x=w556, y=w558) -> (x+y=w557:dbl)
              n193 = Bundle By Name(cluster=w559, "Start X"=w553, "Start Z"=w557, "Specific Arguments"=w549) -> (w547:T1)
              n194 = global write "Trav_pos_global.vi" "Speed Factor"(w548) -> ()
              n195 = call "Set_Traverse_Position.vi"("Currently on Point"=1, "Simulate/Run"=w546, "Traverse line"=w547) -> ("Status Cluster"=w542:T17)  [unwired: 3 in]
              n196 = Unbundle By Name(w542) -> ("Status"=w544:T6)
              n197 = case shown="Default" w544 {
                tunnel: [TRUE TRUE TRUE FALSE] -> w543
                tunnel: [w560 w562 w564 Auto_Calib_Case."Reset Traverse positions" ("Currently in Case")] -> w541
                tunnel: w540 -> [w560 w562 w564 _]
                frame "Continue" {
                }
                frame "Jump to Next Point" {
                }
                frame "Continue with Error" {
                }
                frame Default {
                }
              }
            }
            n198 = call "Merge_Status_Clusters.vi"("Status Cluster 2"=w521, "Status Cluster 1"=w523) -> ("Status Cluster Out"=w522:T17)
          }
          frame #4 {
            n199 = case shown="\"Run VI\"" w573 {
              frame "Check VI only", Default {
              }
              frame "Run VI" {
                n200 = while {
                  shift-right: [w585] -> _
                  shift-left: _ -> [w586]
                  tunnel: [w584] -> w579
                  stop <- TRUE stop-if-true
                  n201 = Get Date/Time In Seconds() -> (seconds since 1Jan1904=w585:timestamp)
                  n202 = Subtract(x=w585, y=w586) -> (x-y=w584:dbl)
                }
                n203 = Divide(x=w579, y=3600.0) -> (x/y=w578:dbl)
                n204 = Multiply(x=w578, y=0.2) -> (x*y=w576:dbl)
                n205 = Add(x=w576, y=0.8) -> (x+y=w574:dbl)
                n206 = In Range and Coerce(upper limit=2.0, x=w574, lower limit=1.0) -> (coerced(x)=→"Wait factor":dbl)  [unwired: 1 out]
              }
            }
            n207 = global write "Trav_pos_global.vi" "Speed Factor"(1.0 ("Speed Factor")) -> ()
          }
        }
      }
      frame "Are There Enough Calibration Points" {
        n208 = Array Size(array=w595) -> (size(s)=w596:i32[])
        n209 = Index Array(array=w596, index=0 ("Index")) -> (element=w590:i32)
        "No of Calib Points" <- w590
        n210 = case shown="2, Default" w590 {
          tunnel: [w599 Auto_Calib_Case."End" ("Currently in Case")] -> w592
          tunnel: w591 -> [w599 _]
          tunnel: w589 -> [w598 w602]
          tunnel: [w598 w601] -> w588
          frame 2, Default {
          }
          frame 0, 1 {
            n211 = Bundle By Name(cluster=w602, "Error Description"="Less than two calibration points have been specified\n", "Status"=Multi_Run_Status."Jump to Next Row") -> (w604:T17)
            n212 = call "Merge_Status_Clusters.vi"("Status Cluster 2"=w604, "Status Cluster 1"=w602) -> ("Status Cluster Out"=w601:T17)
          }
        }
        "Currently On" <- 1 ("Currently On")
      }
      frame "Set Measurement Conditions" {
        n213 = local read "Currently On"() -> (w618:i32)
        n214 = Decrement(x=w618) -> (x-1=w622:i32)
        n215 = Index Array(array=w623, index (row)=w622) -> (element=w621:dbl[])  [unwired: 1 in]
        n216 = case shown="\"Concentration\"" w619 {
          tunnel: w621 -> [w658 _ w680 w691]
          tunnel: w609 -> [_ _ _ _]
          tunnel: w624 -> [w656 w671 w676 w693]
          tunnel: [w657 w671 w675 w689] -> w617
          tunnel: w618 -> [w653 _ _ _]
          tunnel: [0.0 ("f") 0.0 ("f") 5.0 ("f") 0.0] -> w616
          tunnel: [FALSE FALSE FALSE w684] -> w607
          tunnel: w606 -> [_ _ _ w684]
          frame "Tunnel Speed" {
            n217 = Index Array(array=w658, index=0 ("Index")) -> (element=w646:dbl)
            n218 = while {
              shift-right: [w666] -> w648
              shift-left: _ -> [w668]
              tunnel: w646 -> [w667]
              tunnel: [w666] -> w655
              tunnel: [w668] -> w654
              stop <- FALSE continue-if-true
              n219 = Greater?(x=w667, y=-0.5) -> (0:w666:bool)
            }
            n220 = Exclusive Or(1:w654, 2:w655) -> (0:w651:bool)
            n221 = Greater?(x=w653, y=1) -> (0:w650:bool)
            n222 = case shown="False" w648 {
              tunnel: [w660 w662] -> w647
              tunnel: w646 -> [w661 w662]
              frame False {
                n223 = Negate(x=w661) -> (-x=w660:dbl)
              }
              frame True {
              }
            }
            n224 = And(x=w651, y=w650) -> (x .and. y?=w649:bool)
            n225 = case shown="True" w649 {
              frame False {
              }
              frame True {
                n226 = call "Wait_Seconds_with_display.vi"("Message"="Please rotate the probe you are calibrating", "Seconds to wait"=10000.0) -> ()  [unwired: 2 out]
              }
            }
            n227 = Bundle By Name(cluster=w656, "Tunnel Speed"=w647) -> (w657:T1)
          }
          frame "ESC RPM" {
          }
          frame "Traverse Position" {
            n228 = Index Array(array=w680, index=2 ("Index")) -> (element=w677:dbl)
            n229 = Index Array(array=w680, index=0 ("Index")) -> (element=w679:dbl)
            n230 = Index Array(array=w680, index=1 ("Index")) -> (element=w678:dbl)
            n231 = Bundle By Name(cluster=w676, "Start X"=w679, "Start Y"=w678, "Start Z"=w677) -> (w675:T1)
          }
          frame "Concentration" {
            w692 = nan ("Start X")
            # "#Unused Different for cal?"
            n232 = Index Array(array=w691) -> (element #1=w685:dbl, element #2=w686:dbl, element #3=w687:dbl)  [unwired: 3 in]
            "Trace Gas %" <- w687
            n233 = Bundle By Name(cluster=w693, "Start X"=w692, "Start Y"=w692, "Start Z"=w692) -> (w690:T1)
            n234 = Bundle By Name(cluster=w690, "Carrier_1 Q (l/min)"=w685, "Carrier_2 Q (l/min)"=w686, "Trace Gas Concentration (%)"=w687) -> (w689:T1)
          }
        }
        n235 = stacked-sequence {
          tunnel: w609 -> [w629 _]
          tunnel: w617 -> [w628 _]
          tunnel: [w627 _] -> w614
          tunnel: w608 -> [w626 _]
          tunnel: w616 -> [_ w632]
          tunnel: w609 -> [_ w631]
          tunnel: w607 -> [_ _]
          frame #0 {
            n236 = call "Set_Measurement_Conditions.vi"("Traverse line"=w628, "Gas Line Name"=w626, "Currently on Point"=1, "Simulate/Run"=w629, "Source Establishment Time (s)"=5.0) -> ("Status Cluster"=w627:T17)  [unwired: 2 in]
          }
          frame #1 {
            n237 = case shown="\"Run VI\"" w631 {
              tunnel: w632 -> [_ w634]
              frame "Check VI only" {
              }
              frame "Run VI" {
                n238 = call "Wait_Seconds_with_display.vi"("Message"="Establishing Calibration Conditions", "Seconds to wait"=w634) -> ()  [unwired: 1 in, 1 out]
              }
            }
          }
        }
        n239 = call "Merge_Status_Clusters.vi"("Status Cluster 2"=w614, "Status Cluster 1"=w615) -> ("Status Cluster Out"=w613:T17)
        n240 = Unbundle By Name(w613) -> ("Status"=w612:T6)
        n241 = case shown="\"Continue\", \"Continue with Error\"" w612 {
          tunnel: w611 -> [w636 w637 _]
          tunnel: [w635 w638 Auto_Calib_Case."End" ("Currently in Case")] -> w610
          tunnel: w609 -> [_ w639 _]
          frame "Jump to Next Point" {
            n242 = Increment(x=w636) -> (x+1=w635:T7)
          }
          frame "Continue", "Continue with Error" {
            n243 = case shown="\"Run VI\"" w639 {
              tunnel: [w640 w642] -> w638
              tunnel: w637 -> [w641 w642]
              frame "Check VI only" {
                n244 = Increment(x=w641) -> (x+1=w640:T7)
              }
              frame "Run VI" {
              }
            }
          }
          frame "Jump to Next Row", Default {
          }
        }
      }
      frame "Measure Calibration Point" {
        n245 = case shown="\"Concentration\"" w708 {
          tunnel: w707 -> [_ w723 w1049]
          tunnel: [w710 w722 w1048] -> w700
          tunnel: [w711 w721 w1047] -> w704
          tunnel: w703 -> [_ w720 w1046]
          tunnel: [w709 w719 w1045] -> w698
          tunnel: w699 -> [w709 w718 w1044]
          tunnel: w697 -> [_ w717 w1043]
          tunnel: w696 -> [_ _ w1042]
          tunnel: w695 -> [_ _ w1041]
          tunnel: w694 -> [_ w716 _]
          frame "Tunnel Speed", Default {
            n246 = local read "New Calib Filenames"() -> (w713:path[])
            n247 = Index Array(array=w713, index=0 ("Index")) -> (element=w714:path)
            n248 = call "Calibration.vi"("Mode"=Calib_mode."Take a New Calibration Point", "Calib file"=w714) -> ("Coefficients"=w711:dbl[][], "Status Out"=w710:T6)  [unwired: 1 in, 15 out]
          }
          frame "Concentration" {
            # "St Dev"
            # "Mean"
            n249 = stacked-sequence {
              seq-local: [_ w730 _ _] -> [_ _ w959 _]
              seq-local: [_ w729 _ _] -> [_ _ w958 _]
              seq-local: [_ w728 _ _] -> [_ _ w957 _]
              seq-local: [_ _ w956 _] -> [_ _ _ w1025]
              seq-local: [_ _ w954 _] -> [_ _ _ _]
              seq-local: [_ w726 _ _] -> [_ _ w947 _]
              tunnel: w723 -> [_ w733 _ _]
              tunnel: [_ w731 _ _] -> w722
              tunnel: [_ _ w960 _] -> w721
              tunnel: w720 -> [_ _ w955 w1031]
              tunnel: [_ _ _ w1019] -> w719
              tunnel: w718 -> [_ _ _ w1018]
              tunnel: w717 -> [_ _ _ _]
              tunnel: w716 -> [_ _ w948 _]
              frame #0 {
                n250 = global write "Meas_global.vi" "Remote control"(TRUE ("Remote control")) -> ()
                n251 = global write "Meas_global.vi" "Raw data option"(enum16{"Save raw data", "Raw data not saved"}."Save raw data" ("Raw data option")) -> ()
              }
              frame #1 {
                n252 = local read "New Calib Filenames"() -> (w734:path[])
                n253 = local read "HFR500 Comms Channels"() -> (w727:i32[])
                n254 = Index Array(array=w734, index=0 ("Index")) -> (element=w732:path)
                n255 = while {
                  tunnel: [w747] -> w731
                  tunnel: w732 -> [w746]
                  tunnel: w733 -> [w744]
                  tunnel: [w740] -> w730
                  tunnel: [w739] -> w729
                  tunnel: [w742] -> w728
                  tunnel: w727 -> [w741]
                  shift-right: [w737] -> _
                  shift-left: _ -> [w738]
                  tunnel: [w736] -> w726
                  i -> [w743]
                  stop <- w745 continue-if-true
                  # "St Dev"
                  # "Mean"
                  n256 = stacked-sequence {
                    seq-local: [_ w751 _ _ _ _ _ _ _] -> [_ _ _ _ w822 _ _ _ _]
                    seq-local: [_ _ w761 _ _ _ _ _ _] -> [_ _ _ _ w807 _ w843 _ _]
                    seq-local: [_ _ w759 _ _ _ _ _ _] -> [_ _ _ _ w810 _ _ _ w920]
                    seq-local: [_ _ _ _ w813 _ _ _ _] -> [_ _ _ _ _ _ w849 _ _]
                    seq-local: [_ _ w758 _ _ _ _ _ _] -> [_ _ _ _ w809 _ w846 _ w921]
                    seq-local: [_ _ _ _ w806 _ _ _ _] -> [_ _ _ _ _ _ _ _ w916]
                    seq-local: [_ _ _ _ w801 _ _ _ _] -> [_ _ _ _ _ w831 _ _ _]
                    tunnel: [_ w751 _ _ _ _ _ _ _] -> w747
                    tunnel: w746 -> [_ w755 _ _ _ _ w848 _ _]
                    tunnel: [_ _ _ _ w801 _ _ _ _] -> w745
                    tunnel: w744 -> [_ w752 _ _ _ _ _ _ _]
                    tunnel: w743 -> [_ _ _ _ w824 _ _ _ w924]
                    tunnel: [_ w749 _ _ _ _ _ _ _] -> w742
                    tunnel: w741 -> [_ _ _ _ _ _ w847 _ _]
                    tunnel: [_ _ _ _ _ _ w845 _ _] -> w740
                    tunnel: [_ _ _ _ _ _ w844 _ _] -> w739
                    tunnel: w738 -> [_ _ _ _ _ _ _ w910 w917]
                    tunnel: [_ _ _ _ _ _ _ _ w919] -> w737
                    tunnel: [_ _ _ w779 _ _ _ _ _] -> w736
                    frame #0 {
                      n257 = global write "Meas_global.vi" "Remote control"(TRUE ("Remote control")) -> ()
                    }
                    frame #1 {
                      n258 = call "Get_Data_Base_file_code.vi"("Data Type"="Raw_Calibrations", "Results Filename"=w755, "Short_Name"="Raw_Cal" ("Data Type")) -> ("Raw Data File Name"=w749:path)  [unwired: 1 in, 3 out]
                      n259 = call "Measurement.vi"("setup"=Setup."Run Program", "Post Process"=Post_Process."Take New Data", "File"=Save_Data."Save No Data", "Raw data file"=w749, "Setup filename"=w752) -> ("Status Out"=w751:T6)  [unwired: 1 in, 13 out]
                    }
                    frame #2 {
                      n260 = global read "Meas_global.vi" "Time Trace"() -> (w760:T29[])
                      n261 = local read "FF Indexes"() -> (w762:i16[])
                      n262 = for {
                        tunnel: w762 -> [w764] mode=indexing
                        tunnel: [w777] -> w758 mode=indexing
                        tunnel: [w776] -> w761 mode=indexing
                        tunnel: w760 -> [w774]
                        tunnel: [w768] -> w759 mode=indexing
                        n263 = Index Array(array=w774, index=w764) -> (element=w773:T29)
                        n264 = Unbundle By Name(w773) -> ("Eng Values"=w767:dbl[])
                        n265 = call "Get Time Trace.vi"("Channel Index"=w764) -> ("Time (s)"=w763:dbl[])  [unwired: 1 out]
                        n266 = call-poly <vilib>:"Mean.vi"("X"=w767) -> ("mean"=w771:dbl)  [unwired: 1 out]
                        n267 = Divide(x=w763, y=60.0) -> (x/y=w766:dbl[])
                        n268 = Max & Min(x=w771, y=0.3) -> (max(x,y)=w769:dbl)  [unwired: 1 out]
                        n269 = Divide(x=w767, y=w769) -> (x/y=w772:dbl[])
                        n270 = call <vilib>:"Linear Fit.vi"("Y"=w772, "X"=w766) -> ("slope"=w768:dbl)  [unwired: 9 in, 4 out]
                        n271 = call "De-spiked_Stats.vi"("Raw Signal"=w767, "No of st dev to chop at"=6.0) -> ("mean"=w777:dbl, "standard deviation"=w776:dbl)  [unwired: 1 out]
                      }
                    }
                    frame #3 {
                      n272 = global read "Meas_global.vi" "Analysis Info cluster"() -> (w781:T30[])
                      n273 = local read "FF Indexes"() -> (w780:i16[])
                      n274 = call "Black box desired channels.vi"() -> ("Names"=w778:string[])  [unwired: 4 in, 1 out]
                      n275 = for {
                        tunnel: w781 -> [w789]
                        tunnel: w780 -> [w788] mode=indexing
                        tunnel: w778 -> [w785]
                        tunnel: [w784] -> w779 mode=indexing
                        n276 = Index Array(array=w789, index=w788) -> (element=w787:T30)
                        n277 = Unbundle By Name(w787) -> ("Metadata Ch Names"=w783:string[], "Metadata Ch Values"=w786:string[])
                        n278 = for {
                          tunnel: w783 -> [w791] mode=indexing
                          tunnel: [w790] -> w782 mode=indexing
                          n279 = Reverse String(1:w791) -> (0:w794:string)
                          n280 = Match Pattern(string=w794, regular expression=":") -> (before substring=w792:string)  [unwired: 1 in, 3 out]
                          n281 = Reverse String(1:w792) -> (0:w790:string)
                        }
                        n282 = for {
                          tunnel: w782 -> [w800]
                          tunnel: w786 -> [w798]
                          tunnel: w785 -> [w796] mode=indexing
                          tunnel: [w795] -> w784 mode=indexing
                          n283 = Search 1D Array(1D array=w800, element=w796) -> (index of element=w799:i32)  [unwired: 1 in]
                          n284 = Index Array(array=w798, index=w799) -> (element=w797:string)
                          n285 = Fract/Exp String To Number(string=w797) -> (number=w795:dbl)  [unwired: 3 in, 1 out]
                        }
                      }
                    }
                    frame #4 {
                      n286 = for {
                        tunnel: w809 -> [w830] mode=indexing
                        tunnel: [w826] -> w803 mode=indexing
                        n287 = Divide(x=w830, y=3.0) -> (x/y=w828:dbl)
                        n288 = Max & Min(x=w828, y=1.0) -> (max(x,y)=w826:dbl)  [unwired: 1 out]
                      }
                      n289 = Absolute Value(x=w810) -> (abs(x)=w805:dbl[])
                      n290 = Divide(x=w805, y=w803) -> (x/y=w804:dbl[])
                      n291 = Divide(x=w807, y=w803) -> (x/y=w806:dbl[])
                      n292 = Greater?(x=w804, y="Slope less than") -> (0:w820:bool[])
                      n293 = Greater?(x=w806, y="St Dev less than") -> (0:w825:bool[])
                      n294 = Or Array Elements(Boolean array=w820) -> (logical OR=w819:bool)
                      n295 = local read "Multi FFID Range"() -> (w812:bool)
                      n296 = Or Array Elements(Boolean array=w825) -> (logical OR=w818:bool)
                      n297 = Less?(x=w824, y=11) -> (x < y?=w816:bool)
                      n298 = Equal?(x=w822, y=Multi_Run_Status."Continue" ("Status Out")) -> (x = y?=w815:bool)
                      n299 = Or(x=w819, y=w818) -> (x .or. y?=w817:bool)
                      n300 = And(x=w817, y=w816) -> (x .and. y?=w814:bool)
                      n301 = local read "stop"() -> (w802:bool)
                      n302 = Compound Arithmetic op=AND(invert w802, w815, w814) -> (w801:bool)
                      n303 = Compound Arithmetic op=AND(w815, invert w814, w812) -> (w813:bool)
                    }
                    frame #5 {
                      n304 = case shown="True" w831 {
                        frame False {
                        }
                        frame True {
                          n305 = global read "Meas_global.vi" "Raw data file"() -> (w835:path)
                          n306 = Strip Path(path=w835) -> (stripped path=w842:path, name=w838:string)
                          n307 = Strip Path(path=w842) -> (stripped path=w841:path)  [unwired: 1 out]
                          n308 = Build Path(base path=w841, name or relative path="Rejected Raw Data") -> (appended path=w839:path)
                          n309 = Build Path(base path=w839, name or relative path=w838) -> (appended path=w837:path)
                          n310 = call "Create_directory_path.vi"("Dialog Box"=FALSE, "Path name"=w837) -> ("error out"=w833:errorcluster, "Path name Out"=w834:path)  [unwired: 1 in]
                          n311 = Move(source path=w835, error in=w833, 9:TRUE ("overwrite (F)"), 10:w834) -> ()  [unwired: 1 in, 3 out]
                        }
                      }
                    }
                    frame #6 {
                      n312 = case shown="True" w849 {
                        tunnel: w848 -> [_ w857]
                        tunnel: w847 -> [_ w856]
                        tunnel: w846 -> [w851 w855]
                        tunnel: [w851 w854] -> w845
                        tunnel: [w850 w852] -> w844
                        tunnel: w843 -> [w850 w853]
                        frame False {
                        }
                        frame True {
                          n313 = stacked-sequence {
                            tunnel: w857 -> [_ _ w870 _ _]
                            tunnel: w856 -> [w862 _ _ _ w896]
                            tunnel: w855 -> [_ _ _ w882 _]
                            tunnel: [_ _ _ w880 _] -> w854
                            tunnel: w853 -> [_ _ _ w879 _]
                            tunnel: [_ _ _ w878 _] -> w852
                            frame #0 {
                              n314 = global write "Meas_global.vi" "Remote control"(TRUE ("Remote control")) -> ()
                              n315 = for {
                                tunnel: w862 -> [w868] mode=indexing
                                tunnel: "High Range ppm" -> [w867]
                                shift-right: [w864] -> w859
                                shift-left: errorcluster {"status"=FALSE, "code"=0, "source"=""} ("error IO") -> [w865]
                                n316 = call "HFR500 Set Range.vi"("Ch number"=w868, "ppm Range"=w867) -> ("error out"=w866:errorcluster)  [unwired: 2 out]
                                n317 = Merge Errors(w866, w865) -> (w864:errorcluster)
                              }
                              n318 = call "EnFlo_Error_Handler.vi"("error in (no error)"=w859, "Error Type"="HFR500 Set Range") -> ()  [unwired: 2 in, 2 out]
                            }
                            frame #1 {
                              n319 = Wait (ms)(milliseconds to wait=u32 2000) -> ()  [unwired: 1 out]
                            }
                            frame #2 {
                              n320 = call "Get_Data_Base_file_code.vi"("Data Type"="Raw_Calibrations", "Results Filename"=w870, "Short_Name"="Raw_Cal" ("Data Type")) -> ("Raw Data File Name"=w876:path)  [unwired: 1 in, 3 out]
                              n321 = call "Measurement.vi"("setup"=Setup."Run Program", "Post Process"=Post_Process."Take New Data", "File"=Save_Data."Save No Data", "Raw data file"=w876) -> ()  [unwired: 2 in, 14 out]
                            }
                            frame #3 {
                              n322 = global read "Meas_global.vi" "Time Trace"() -> (w883:T29[])
                              n323 = local read "FF Indexes"() -> (w884:i16[])
                              n324 = for {
                                tunnel: w884 -> [w891] mode=indexing
                                tunnel: [w890] -> w881 mode=indexing
                                tunnel: [w889] -> w877 mode=indexing
                                tunnel: w883 -> [w887]
                                n325 = Index Array(array=w887, index=w891) -> (element=w886:T29)
                                n326 = Unbundle By Name(w886) -> ("Eng Values"=w885:dbl[])
                                n327 = call "De-spiked_Stats.vi"("Raw Signal"=w885, "No of st dev to chop at"=6.0) -> ("mean"=w890:dbl, "standard deviation"=w889:dbl)  [unwired: 1 out]
                              }
                              n328 = Build Array (concatenate)(w882, w881) -> (w880:dbl[])
                              n329 = Build Array (concatenate)(w879, w877) -> (w878:dbl[])
                            }
                            frame #4 {
                              n330 = for {
                                tunnel: w896 -> [w901] mode=indexing
                                tunnel: HFR500_ppm_Range."1,000" ("High Range ppm 2") -> [w900]
                                shift-right: [w897] -> w894
                                shift-left: errorcluster {"status"=FALSE, "code"=0, "source"=""} ("error IO") -> [w898]
                                n331 = call "HFR500 Set Range.vi"("Ch number"=w901, "ppm Range"=w900) -> ("error out"=w899:errorcluster)  [unwired: 2 out]
                                n332 = Merge Errors(w899, w898) -> (w897:errorcluster)
                              }
                              n333 = call "EnFlo_Error_Handler.vi"("error in (no error)"=w894, "Error Type"="HFR500 Set Range") -> ()  [unwired: 2 in, 2 out]
                            }
                          }
                        }
                      }
                    }
                    frame #7 {
                      w902 = 11 ("y")
                      w906 = 1 ("index")
                      n334 = Array Size(array=w910) -> (size(s)=w909:i32[])
                      n335 = Index Array(array=w909, index=w906) -> (element=w903:i32)
                      n336 = Less?(x=w903, y=w902) -> (x < y?=w905:bool)
                      n337 = property on="Calib Repeats" class="Arr (strict)"() -> ("Index Values"=w908:u32[])  [unwired: 2 in, 2 out]
                      n338 = case shown="False" w905 {
                        tunnel: [w911 u32 0 ("new element/subarray")] -> w904
                        tunnel: w903 -> [w914 _]
                        tunnel: w902 -> [w913 _]
                        frame False {
                          n339 = Subtract(x=w914, y=w913) -> (x-y=w912:i32)
                          n340 = To Unsigned Long Integer(number=w912) -> (unsigned 32bit integer=w911:u32)
                        }
                        frame True {
                        }
                      }
                      n341 = Replace Array Subset(array=w908, new element=w904, index=w906) -> (w907:u32[])
                      n342 = property on="Calib Repeats" class="Arr (strict)"("Index Values"=w907) -> ()  [unwired: 2 in, 2 out]
                    }
                    frame #8 {
                      n343 = local read "Currently On"() -> (w926:i32)
                      n344 = Equal To 0?(x=w924) -> (x = 0?=w922:bool)
                      n345 = Equal?(x=w926, y=1) -> (x = y?=w923:bool)
                      n346 = And(x=w923, y=w922) -> (x .and. y?=w918:bool)
                      n347 = case shown="False" w918 {
                        tunnel: w921 -> [w930 w940]
                        tunnel: w916 -> [w929 w939]
                        tunnel: w920 -> [w928 w938]
                        tunnel: [w927 w937] -> w919
                        tunnel: w917 -> [_ w936]
                        frame True {
                          n348 = for {
                            tunnel: w930 -> [w935] mode=indexing
                            tunnel: w929 -> [w934] mode=indexing
                            tunnel: w928 -> [w933] mode=indexing
                            tunnel: [w931] -> w927 mode=indexing
                            n349 = Build Array(w935, w934, w933) -> (w932:dbl[])
                            n350 = Build Array(w932) -> (w931:dbl[][])
                          }
                        }
                        frame False {
                          n351 = for {
                            tunnel: w940 -> [w946] mode=indexing
                            tunnel: w939 -> [w945] mode=indexing
                            tunnel: w938 -> [w944] mode=indexing
                            tunnel: [w942] -> w937 mode=indexing
                            tunnel: w936 -> [w941] mode=indexing
                            n352 = Build Array(w946, w945, w944) -> (w943:dbl[])
                            n353 = Build Array (concatenate)(w941, w943) -> (w942:dbl[][])
                          }
                        }
                      }
                      "Calib Repeats" <- w919
                    }
                  }
                }
              }
              frame #2 {
                n354 = local read "FFID St Dev"() -> (w962:dbl[][])
                n355 = Build Array (concatenate)(w959, w958) -> (w961:dbl[])
                n356 = call "Read_RD_Ch_header.vi"("Raw data file"=w957) -> ("Ch Name Out"=w950:string[], "Ch Values"=w949:string[])  [unwired: 2 out]
                n357 = case shown="\"GMU1 Source\", Default" w948 {
                  tunnel: [w965 w975 w997] -> w956
                  tunnel: [nan nan w996] -> w954
                  tunnel: w955 -> [_ _ w995]
                  tunnel: [0.0 ("t") 0.0 ("t") w994] -> w951
                  tunnel: w950 -> [w974 w982 w992]
                  tunnel: w949 -> [w973 w981 w991]
                  frame "GMU2 Source" {
                    n358 = Search 1D Array(1D array=w974, element="GMU2:Source:Meas Strength") -> (index of element=w971:i32)  [unwired: 1 in]
                    n359 = Index Array(array=w973, index=w971) -> (element=w970:string)
                    n360 = Fract/Exp String To Number(string=w970) -> (number=w967:dbl)  [unwired: 3 in, 1 out]
                    n361 = Multiply(x=w967, y=10000.0) -> (x*y=w965:dbl)
                  }
                  frame "GMU2 Calib" {
                    n362 = Search 1D Array(1D array=w982, element="GMU2:Calib:Meas ppm") -> (index of element=w979:i32)  [unwired: 1 in]
                    n363 = Index Array(array=w981, index=w979) -> (element=w978:string)
                    n364 = Fract/Exp String To Number(string=w978) -> (number=w975:dbl)  [unwired: 3 in, 1 out]
                  }
                  frame "GMU1 Source", Default {
                    n365 = Search 1D Array(1D array=w992, element="GMU:Source:ppm/%Density") -> (index of element=w984:i32)  [unwired: 1 in]
                    n366 = Search 1D Array(1D array=w992, element="GMU:Source:Meas Strength") -> (index of element=w987:i32)  [unwired: 1 in]
                    n367 = Index Array(array=w991, index=w984) -> (element=w985:string)
                    n368 = Index Array(array=w991, index=w987) -> (element=w986:string)
                    n369 = Fract/Exp String To Number(string=w985) -> (number=w996:dbl)  [unwired: 3 in, 1 out]
                    n370 = Fract/Exp String To Number(string=w986) -> (number=w993:dbl)  [unwired: 3 in, 1 out]
                    n371 = Not A Number/Path/Refnum?(number/path/refnum=w996) -> (NaN/Path/Refnum?=w990:bool)
                    n372 = Select(t=0.0, s=w990, f=w996) -> (s? t:f=w994:dbl)
                    n373 = Multiply(x=w995, y=w993) -> (x*y=w997:dbl)
                  }
                }
                n374 = Build Array (concatenate)(w962, w961) -> (→"FFID St Dev":dbl[][])
                n375 = local read "New Calib Filenames"() -> (w964:path[])
                n376 = for {
                  tunnel: w959 -> [w1004] mode=indexing
                  tunnel: w956 -> [w1003]
                  tunnel: [w1002] -> w960 mode=indexing
                  tunnel: w964 -> [w1001] mode=indexing
                  tunnel: w958 -> [w1000] mode=indexing
                  tunnel: w954 -> [w999]
                  tunnel: w947 -> [w998] mode=indexing
                  n377 = stacked-sequence {
                    tunnel: w1004 -> [w1012 _]
                    tunnel: w1003 -> [w1011 _]
                    tunnel: [_ w1014] -> w1002
                    tunnel: w1001 -> [_ w1013]
                    tunnel: w1000 -> [w1009 _]
                    tunnel: w999 -> [w1008 _]
                    tunnel: w998 -> [w1006 _]
                    frame #0 {
                      n378 = global read "Meas_global.vi" "Temp"() -> (w1007:dbl)
                      n379 = Build Array (concatenate)(w1011, w1012, w1009, w1008, w1007, 1.0, w1006) -> (w1010:dbl[])
                      n380 = global write "Calib_global.vi" "Calibration Points"(w1010) -> ()
                    }
                    frame #1 {
                      n381 = call "Calibration.vi"("Mode"=Calib_mode."Refit Curve", "Calib file"=w1013) -> ("Coefficients"=w1015:dbl[][])  [unwired: 1 in, 16 out]
                      n382 = Index Array(array=w1015, index (row)=0 ("Index")) -> (element=w1014:dbl[])  [unwired: 1 in]
                    }
                  }
                }
                n383 = local read "ppm/%Density"() -> (w952:dbl[])
                n384 = Build Array (concatenate)(w952, w951) -> (→"ppm/%Density":dbl[])
              }
              frame #3 {
                n385 = local read "Trace Gas %"() -> (w1030:dbl)
                n386 = local read "Currently On"() -> (w1024:i32)
                n387 = Multiply(x=w1031, y=w1030) -> (x*y=w1026:dbl)
                n388 = Equal?(x=1, y=w1024) -> (x = y?=w1021:bool)
                n389 = call "In_Range_check.vi"("±"=50.0, "%"=10.0, "Mode"=In_Range."% & ±", "Value"=w1025, "Setpoint"=w1026) -> ("In Range"=w1022:bool)  [unwired: 2 in]
                n390 = Or(x=w1022, y=w1021) -> (x .or. y?=w1020:bool)
                n391 = case shown="False" w1020 {
                  tunnel: w1026 -> [w1039 _]
                  tunnel: w1025 -> [w1038 _]
                  tunnel: [w1032 w1040] -> w1019
                  tunnel: w1018 -> [w1033 w1040]
                  frame False {
                    n392 = Format Into String(format string="Error in Mixing Calibration Gas\nDemanded %.0fppm, Measured %.0fppm.", w1039, w1038) -> (resulting string=w1034:string)  [unwired: 2 in, 1 out]
                    n393 = Bundle By Name(cluster=w1033, "Error Description"=w1034, "Status"=Multi_Run_Status."Jump to Next Point") -> (w1036:T17)
                    n394 = call "Merge_Status_Clusters.vi"("Status Cluster 2"=w1036, "Status Cluster 1"=w1033) -> ("Status Cluster Out"=w1032:T17)
                  }
                  frame True {
                  }
                }
              }
            }
          }
          frame "ESC RPM" {
            # "PWM"
            # "RPM"
            n395 = stacked-sequence {
              seq-local: [w1051 _ _ _] -> [_ _ _ w1073]
              seq-local: [_ _ w1066 _] -> [_ _ _ w1072]
              tunnel: w1049 -> [_ _ _ _]
              tunnel: [_ _ _ w1075] -> w1048
              tunnel: [_ _ _ w1077] -> w1047
              tunnel: w1046 -> [_ _ _ _]
              tunnel: [_ _ _ w1074] -> w1045
              tunnel: w1044 -> [_ _ _ w1074]
              tunnel: w1043 -> [_ _ _ _]
              tunnel: w1042 -> [_ w1059 _ _]
              tunnel: w1041 -> [w1055 _ _ _]
              frame #0 {
                n396 = local read "Currently On"() -> (w1054:i32)
                n397 = Decrement(x=w1054) -> (x-1=w1056:i32)
                n398 = Index Array(array=w1055, index (row)=w1056) -> (element=w1053:dbl[])  [unwired: 1 in]
                n399 = Index Array(array=w1053, index=0 ("Index")) -> (element=w1051:dbl)
                n400 = call "ESC controller ramped.vi"("Don't Wait"=FALSE, "Output %"=w1051) -> ("Error out"=w1050:errorcluster)  [unwired: 1 in]
                n401 = call "EnFlo_Error_Handler.vi"("error in (no error)"=w1050) -> ()  [unwired: 3 in, 2 out]
              }
              frame #1 {
                w1063 = ""
                w1062 = FALSE  # Remote control
                n402 = Unbundle By Name(w1059) -> ("Meas Setup File"=w1058:string)
                n403 = call "Code_to_run.vi"("Extra command String"=w1063, "Current Row Comments"=w1063, "setup"=Setup."Run Program", "Remote control"=w1062, "File"=Save_Data."Save No Data", "Results Filename"=path "C:/EDF_Speed_Control.xls", "Averaging time (min)"=0.01, "Setup filename"=w1058) -> ()  [unwired: 4 in, 4 out]
              }
              frame #2 {
                n404 = global read "Dynamic_call_global.ph.vi" "Plug in titles"() -> (w1067:string[])
                n405 = global read "Dynamic_call_global.ph.vi" "Plug in values"() -> (w1069:string[])
                n406 = Search 1D Array(1D array=w1067, element="Aero_Tunnel:EDF:Meas RPM" ("string")) -> (index of element=w1070:i32)  [unwired: 1 in]
                n407 = Index Array(array=w1069, index=w1070) -> (element=w1071:string)
                n408 = Fract/Exp String To Number(string=w1071) -> (number=w1066:dbl)  [unwired: 3 in, 1 out]
              }
              frame #3 {
                n409 = local read "New Calib Filenames"() -> (w1079:path[])
                n410 = Index Array(array=w1079) -> (element=w1078:path)  [unwired: 1 in]
                n411 = stacked-sequence {
                  tunnel: w1072 -> [w1084 _]
                  tunnel: w1073 -> [w1083 _]
                  tunnel: [_ w1086] -> w1076
                  tunnel: w1078 -> [_ w1085]
                  frame #0 {
                    w1080 = 0.0 ("standard deviation")
                    n412 = global read "Meas_global.vi" "Temp"() -> (w1081:dbl)
                    n413 = Build Array(w1083, w1084, w1080, w1080, w1081) -> (w1082:dbl[])
                    n414 = global write "Calib_global.vi" "Calibration Points"(w1082) -> ()
                  }
                  frame #1 {
                    n415 = call "Calibration.vi"("Mode"=Calib_mode."Refit Curve", "Calib file"=w1085) -> ("Coefficients"=w1087:dbl[][])  [unwired: 1 in, 16 out]
                    n416 = Index Array(array=w1087, index (row)=0 ("Index")) -> (element=w1086:dbl[])  [unwired: 1 in]
                  }
                }
                n417 = Build Array(w1076) -> (w1077:dbl[][])
                n418 = global read "Meas_global.vi" "Status"() -> (w1075:T6)
              }
            }
          }
        }
        "Coefficients" <- w704
        n419 = Bundle By Name(cluster=w698, "Status"=w700) -> (w702:T17)
        n420 = call "Merge_Status_Clusters.vi"("Status Cluster 2"=w702, "Status Cluster 1"=w698) -> ("Status Cluster Out"=w701:T17)
      }
      frame "Do Another Calibration Point?" {
        n421 = Unbundle By Name(w1090) -> ("Status"=w1092:T6)
        n422 = case shown="\"Terminate Run\"" w1092 {
          tunnel: [w1116 w1117 w1118 TRUE TRUE w1123] -> w1101
          tunnel: [w1116 w1117 w1118 FALSE FALSE w1123] -> w1102
          frame "Continue" {
            w1116 = TRUE
          }
          frame "Continue with Error" {
            w1117 = TRUE
          }
          frame "Jump to Next Point" {
            w1118 = TRUE
          }
          frame "Jump to Next Row" {
          }
          frame "Jump To Fall Back" {
          }
          frame "Terminate Run" {
            w1123 = FALSE
          }
        }
        n423 = local read "No of Calib Points"() -> (w1103:i32)
        n424 = local read "Currently On"() -> (w1096:i32)
        n425 = Greater?(x=w1103, y=w1096) -> (0:w1100:bool)
        n426 = Compound Arithmetic op=AND(invert "stop", w1101) -> (w1099:bool)
        n427 = case shown="True" "stop" {
          tunnel: [w1104 w1107] -> w1091
          tunnel: w1090 -> [w1104 w1108]
          frame False {
          }
          frame True {
            n428 = Bundle By Name(cluster=w1108, "Error Description"="Stop Button Pressed", "Status"=Multi_Run_Status."Terminate Run") -> (w1107:T17)
          }
        }
        n429 = Compound Arithmetic op=AND(w1099, w1102, w1100) -> (w1097:bool)
        n430 = case shown="False" w1097 {
          tunnel: w1096 -> [_ w1115]
          tunnel: [w1109 Auto_Calib_Case."Set Measurement Conditions" ("Currently in Case")] -> w1095
          tunnel: w1094 -> [w1110 _]
          frame False {
            n431 = case shown="\"Run VI\"" w1110 {
              tunnel: [Auto_Calib_Case."Reset Traverse positions" ("Currently in Case") Auto_Calib_Case."Skip Next Frame?" ("Currently in Case")] -> w1109
              frame "Check VI only" {
              }
              frame "Run VI" {
              }
            }
          }
          frame True {
            n432 = Increment(x=w1115) -> (x+1=w1114:i32)
            n433 = local write "Currently On"(w1114) -> ()
          }
        }
      }
      frame "Skip Next Frame?" {
        n434 = case shown="\"Concentration\"" w1130 {
          tunnel: w1129 -> [_ w1136]
          tunnel: w1128 -> [_ w1137]
          tunnel: w1125 -> [_ w1135]
          tunnel: w1124 -> [_ w1134]
          frame "Tunnel Speed", Default {
          }
          frame "Concentration" {
            n435 = stacked-sequence {
              tunnel: w1137 -> [_ w1149]
              tunnel: w1136 -> [_ w1148]
              tunnel: w1135 -> [_ w1145]
              tunnel: w1134 -> [w1138 _]
              frame #0 {
                n436 = case shown="True" w1138 {
                  frame False {
                  }
                  frame True {
                    n437 = stacked-sequence {
                      frame #0 {
                        n438 = call "ASYNC_Adam_client.vi"("Values"=dbl[] [0.0], "Channel Names"=string[] ["Clean_Air:Hi-Tec:Dem Volt"]) -> ()  [unwired: 1 in, 2 out]
                      }
                      frame #1 {
                        n439 = call "Wait_Seconds_with_display.vi"("Message"="Shutting down calibration flow", "Seconds to wait"=20.0) -> ()  [unwired: 1 in, 1 out]
                      }
                    }
                  }
                }
              }
              frame #1 {
                w1143 = 0.0 ("Carrier_1 Q (l/min)")
                n440 = Bundle By Name(cluster=w1149, "Carrier_1 Q (l/min)"=w1143, "Carrier_2 Q (l/min)"=w1143, "Trace Gas Concentration (%)"=w1143) -> (w1147:T1)
                n441 = call "Set_Source.vi"("Source Establishment Time (s)"=0.0, "Source Status"=Client_Source_Status."Not Using", "Gas Line Name"=w1145, "Traverse line"=w1147, "Simulate/Run"=w1148) -> ()  [unwired: 6 out]
              }
            }
          }
        }
        n442 = Unbundle By Name(w1126) -> ("Status"=w1127:T6)
        n443 = case shown="\"Terminate Run\", Default" w1127 {
          tunnel: [w1150 w1151 Auto_Calib_Case."Reset Traverse positions" ("Currently in Case")] -> w1132
          tunnel: w1131 -> [w1150 w1151 _]
          frame "Continue" {
          }
          frame "Continue with Error" {
          }
          frame "Terminate Run", Default {
          }
        }
      }
      frame "Insert New calibration Filenames into Measurement Setup file" {
        n444 = local read "New Calib Filenames"() -> (w1156:path[])
        n445 = local read "Ch No's"() -> (w1153:string[])
        n446 = case shown="\"Concentration\"" w1155 {
          tunnel: [Auto_Calib_Case."Warn if Current Calibration fit is poor" ("Currently in Case") w1168] -> w1160
          tunnel: w1159 -> [_ w1168]
          tunnel: w1156 -> [_ w1167]
          tunnel: [1 w1166] -> w1158
          frame "Tunnel Speed", Default {
          }
          frame "Concentration" {
            n447 = Array Size(array=w1167) -> (size(s)=w1166:i32)
          }
        }
        n448 = call "Current_Calib_Filenames.vi"("Calib Filename"=w1156, "Channel ID input"=w1153, "Mode"=App_Global."Write to Global") -> ()  [unwired: 3 out]
        n449 = global read "Meas_global.vi" "Raw data file"() -> (w1162:path)
        n450 = Strip Path(path=w1162) -> (stripped path=w1161:path)  [unwired: 1 out]
        n451 = for {
          N: w1158 -> [_]
          tunnel: w1156 -> [w1170] mode=indexing
          tunnel: w1161 -> [w1174]
          w1172 = FALSE  # Variable Target?
          n452 = Strip Path(path=w1170) -> (name=w1173:string)  [unwired: 1 out]
          n453 = Build Path(base path=w1174, name or relative path=w1173) -> (appended path=w1169:path)
          n454 = call "Copy_with_Check.vi"("Mode"=enum16{"Move", "Copy"}."Copy", "Target Path"=w1169, "Variable Target?"=w1172, "Source Path"=w1170) -> ()  [unwired: 1 out]
          n455 = call "Remember_Calib_Filenames.vi"("Filename to Remember"=w1169) -> ()  [unwired: 1 out]
        }
      }
      frame "Warn if FFID calibration is very non linear" {
        w1207 = FALSE  # Dialog Box (T)
        n456 = local read "Concentrations"() -> (w1187:dbl[])
        n457 = local read "ppm/%Density"() -> (w1194:dbl[])
        n458 = local read "Clear Calib History"() -> (w1190:bool)
        n459 = Array Max & Min(array=w1187) -> (max value=w1186:dbl)  [unwired: 3 out]
        n460 = Array Subset(array=w1194, index=1) -> (w1192:dbl[])  [unwired: 1 in]
        n461 = feedback #1() -> (w1188:dbl)  [unwired: 1 in]
        n462 = call-poly <vilib>:"Mean.vi"("X"=w1192) -> ("mean"=w1189:dbl)  [unwired: 1 out]
        n463 = feedback-in #1(w1189) -> ()
        n464 = Greater?(x=w1186, y=1500.0) -> (0:w1180:bool)
        n465 = Equal To 0?(x=w1189) -> (x = 0?=w1191:bool)
        n466 = case shown="False" w1190 {
          tunnel: w1189 -> [w1218 _]
          tunnel: w1188 -> [w1217 _]
          frame False {
            n467 = Subtract(x=w1218, y=w1217) -> (x-y=w1216:dbl)
            n468 = Absolute Value(x=w1216) -> (abs(x)=w1215:dbl)
            n469 = Greater?(x=w1215, y=0.5) -> (0:w1213:bool)
            n470 = local write "Clear Calib History"(w1213) -> ()
          }
          frame True {
          }
        }
        n471 = local read "Root Name"() -> (w1206:string[])
        n472 = Select(t=2.2, s=w1191, f=3.9 ("y")) -> (s? t:f=w1184:dbl)
        n473 = Select(t=1.25, s=w1180, f=1.0 ("y")) -> (s? t:f=w1179:dbl)
        n474 = Multiply(x=w1179, y=w1184) -> (x*y=w1183:dbl)
        n475 = local read "Coefficients"() -> (w1209:dbl[][])
        n476 = for {
          tunnel: w1209 -> [w1224] mode=indexing
          shift-right: [w1226] -> w1204
          shift-left: "" -> [w1227]
          tunnel: w1206 -> [w1228] mode=indexing
          tunnel: [w1221] -> w1200 mode=indexing
          tunnel: "If the calibration fit for %s had been linear instead of a second order polynomial, it would have yielded an average fit error of %.1f%%.\\n" ("Format String") -> [w1220]
          tunnel: w1183 -> [w1219]
          n477 = Index Array(array=w1224, index=0 ("Index")) -> (element=w1222:dbl)
          n478 = Absolute Value(x=w1222) -> (abs(x)=w1221:dbl)
          n479 = Less?(x=w1221, y=w1219) -> (x < y?=w1225:bool)
          n480 = case shown="False" w1225 {
            tunnel: w1228 -> [w1230 _]
            tunnel: w1221 -> [w1231 _]
            tunnel: w1227 -> [w1234 w1235]
            tunnel: [w1232 w1235] -> w1226
            tunnel: w1220 -> [w1229 _]
            frame False {
              n481 = Format Into String(format string=w1229, w1230, w1231) -> (resulting string=w1233:string)  [unwired: 2 in, 1 out]
              n482 = Concatenate Strings(w1234, w1233) -> (w1232:string)
            }
            frame True {
            }
          }
        }
        n483 = Array Max & Min(array=w1200) -> (max value=w1199:dbl)  [unwired: 3 out]
        n484 = Empty String/Path?(string/path=w1204) -> (empty?=w1203:bool)
        n485 = Not(x=w1203) -> (.not. x?=w1202:bool)
        n486 = Greater?(x=w1199, y=7.0) -> (0:w1177:bool)
        n487 = case shown="False" w1177 {
          tunnel: ["Poor FFID Linearity" "Very Poor FFID Linearity"] -> w1176
          frame False {
          }
          frame True {
          }
        }
        n488 = Bundle By Name(cluster=errorcluster {"status"=FALSE, "code"=0, "source"=""} ("error in (no error)"), "source"=w1204, "status"=w1202) -> (w1201:errorcluster)
        n489 = call "EnFlo_Error_Handler.vi"("error in (no error)"=w1201, "Error Type"=w1176, "Dialog Box (F)"=w1207) -> ()  [unwired: 3 out]
      }
      frame "Warn if FFID voltages are too low" {
        n490 = local read "Coefficients"() -> (w1245:dbl[][])
        n491 = local read "Concentrations"() -> (w1242:dbl[])
        n492 = Array Max & Min(array=w1242) -> (max value=w1243:dbl)  [unwired: 3 out]
        n493 = local read "New Calib Filenames"() -> (w1244:path[])
        n494 = for {
          shift-right: [w1268] -> w1241
          shift-left: "" -> [w1269]
          tunnel: "For %s the maximum measured calibration voltage was %.1f volts.\nThe Program will now Jump to the next Fall Back Row." ("Format String") -> [w1267]
          tunnel: w1245 -> [w1265] mode=indexing
          tunnel: w1244 -> [w1261] mode=indexing
          tunnel: w1243 -> [w1260]
          n495 = Split 1D Array(array=w1265, index=1) -> (second subarray=w1264:dbl[])  [unwired: 1 out]
          n496 = call "Polybackwards.vi"("Coefficients"=w1264, "Y input"=w1260) -> ("X output"=w1259:dbl)  [unwired: 1 out]
          n497 = Less?(x=w1259, y=0.2) -> (x < y?=w1262:bool)
          n498 = case shown="True" w1262 {
            tunnel: w1269 -> [w1270 w1277]
            tunnel: [w1270 w1275] -> w1268
            tunnel: w1267 -> [_ w1274]
            tunnel: w1261 -> [_ w1273]
            tunnel: w1259 -> [_ w1271]
            frame False {
            }
            frame True {
              n499 = Strip Path(path=w1273) -> (name=w1272:string)  [unwired: 1 out]
              n500 = Format Into String(format string=w1274, w1272, w1271) -> (resulting string=w1276:string)  [unwired: 2 in, 1 out]
              n501 = Concatenate Strings(w1277, w1276) -> (w1275:string)
            }
          }
        }
        n502 = Empty String/Path?(string/path=w1241) -> (empty?=w1240:bool)
        n503 = case shown="False" w1240 {
          tunnel: [w1254 w1258] -> w1238
          tunnel: w1239 -> [w1255 w1258]
          tunnel: w1241 -> [w1252 _]
          tunnel: w1237 -> [w1250 w1257]
          tunnel: [w1249 w1257] -> w1236
          frame False {
            n504 = Bundle By Name(cluster=w1255, "Status"=Multi_Run_Status."Jump To Fall Back", "Error Description"=w1252, "Error Type"="Low FFID calibration voltages") -> (w1256:T17)
            n505 = Increment(x=w1250) -> (x+1=w1249:T7)
            n506 = call "Merge_Status_Clusters.vi"("Status Cluster 2"=w1256, "Status Cluster 1"=w1255) -> ("Status Cluster Out"=w1254:T17)
          }
          frame True {
          }
        }
      }
      frame "Warn if FFID variance is high" {
        w1299 = FALSE  # Dialog Box (T)
        n507 = local read "New Calib Filenames"() -> (w1282:path[])
        n508 = local read "FFID St Dev"() -> (w1301:dbl[][])
        n509 = Index Array(array=w1287, index (col)=0 ("disabled index (col)")) -> (element=w1285:dbl[])  [unwired: 1 in]
        n510 = Array Size(array=w1282) -> (size(s)=w1281:i32)
        n511 = for {
          tunnel: w1301 -> [w1318]
          shift-right: [w1320] -> w1297
          shift-left: "" -> [w1321]
          tunnel: w1282 -> [w1309] mode=indexing
          tunnel: "For %s the measurement at %dppm had a standard deviation of %.2f volts for an average value of  %.1f volts.\\n" ("Format String") -> [w1319]
          tunnel: w1285 -> [w1312]
          tunnel: [w1311] -> w1283 mode=indexing
          tunnel: w1281 -> [w1307]
          tunnel: [w1303] -> w1279 mode=indexing
          i -> [w1306]
          n512 = Strip Path(path=w1309) -> (name=w1308:string)  [unwired: 1 out]
          n513 = Add(x=w1307, y=w1306) -> (x+y=w1305:i32)
          n514 = Index Array(array=w1318, index (col)=w1306) -> (element=w1310:dbl[])  [unwired: 1 in]
          n515 = Index Array(array=w1318, index (col)=w1305) -> (element=w1304:dbl[])  [unwired: 1 in]
          n516 = call-poly <vilib>:"Mean.vi"("X"=w1310) -> ("mean"=w1317:dbl)  [unwired: 1 out]
          n517 = Divide(x=w1304, y=w1317) -> (x/y=w1316:dbl[])
          n518 = Array Max & Min(array=w1304) -> (min value=w1303:dbl)  [unwired: 3 out]
          n519 = Array Max & Min(array=w1316) -> (max value=w1311:dbl, max index (indices)=w1313:i32)  [unwired: 2 out]
          n520 = Greater?(x=w1311, y=0.06) -> (0:w1314:bool)
          n521 = case shown="True" w1314 {
            tunnel: w1308 -> [_ w1332]
            tunnel: w1321 -> [w1322 w1338]
            tunnel: [w1322 w1336] -> w1320
            tunnel: w1319 -> [_ w1335]
            tunnel: w1313 -> [_ w1333]
            tunnel: w1312 -> [_ w1334]
            tunnel: w1304 -> [_ w1331]
            tunnel: w1310 -> [_ w1329]
            frame False {
            }
            frame True {
              n522 = local read "Concentrations"() -> (w1327:dbl[])
              n523 = Index Array(array=w1331, index=w1333) -> (element=w1325:dbl)
              n524 = Index Array(array=w1334, index=w1333) -> (element=w1328:dbl)
              n525 = Index Array(array=w1329, index=w1333) -> (element=w1330:dbl)
              n526 = Index Array(array=w1327, index=w1328) -> (element=w1326:dbl)
              n527 = Multiply(x=w1325, y=2.5) -> (x*y=w1324:dbl)
              n528 = Format Into String(format string=w1335, w1332, w1326, w1324, w1330) -> (resulting string=w1337:string)  [unwired: 2 in, 1 out]
              n529 = Concatenate Strings(w1338, w1337) -> (w1336:string)
            }
          }
        }
        "Minimum St Dev" <- w1279
        n530 = Array Max & Min(array=w1283) -> (max value=w1293:dbl)  [unwired: 3 out]
        n531 = Greater?(x=w1293, y=0.09) -> (0:w1291:bool)
        n532 = Select(t="Very unstable FFID calibration point", s=w1291, f="Unstable FFID calibration point") -> (s? t:f=w1288:string)
        n533 = Empty String/Path?(string/path=w1297) -> (empty?=w1296:bool)
        n534 = Not(x=w1296) -> (.not. x?=w1295:bool)
        n535 = Bundle By Name(cluster=errorcluster {"status"=FALSE, "code"=0, "source"=""} ("error in (no error)"), "source"=w1297, "status"=w1295) -> (w1294:errorcluster)
        n536 = call "EnFlo_Error_Handler.vi"("error in (no error)"=w1294, "Error Type"=w1288, "Dialog Box (F)"=w1299) -> ()  [unwired: 3 out]
      }
      frame "Insert Bkgnd Variance into calib file" {
        n537 = local read "New Calib Filenames"() -> (w1343:path[])
        n538 = local read "Minimum St Dev"() -> (w1344:dbl[])
        n539 = local read "Coefficients"() -> (w1342:dbl[][])
        n540 = for {
          tunnel: w1344 -> [w1348] mode=indexing
          tunnel: w1343 -> [w1354] mode=indexing
          tunnel: w1342 -> [w1351] mode=indexing
          n541 = call "Read_File_Simple.vi"("Filename"=w1354) -> ("string"=w1358:string)  [unwired: 2 in, 7 out]
          n542 = Index Array(array=w1351, index=2) -> (element=w1349:dbl)
          n543 = Multiply(x=w1348, y=w1349) -> (x*y=w1347:dbl)
          n544 = Square(x=w1347) -> (x^2=w1346:dbl)
          n545 = Number To Fractional String(number=w1346, precision (6)=i16 8) -> (F-format string=w1356:string)  [unwired: 2 out]
          n546 = call "Replace_data_in_setup_string.vi"("New data string"=w1356, "Input string"=w1358, "Variable name"="Fast FID Bkgnd Variance") -> ("Appended string"=w1353:string)
          n547 = call "Write_File_Simple.vi"("append to file? (new file:F)"=FALSE, "character string"=w1353, "file path"=w1354) -> ()  [unwired: 2 out]
        }
        n548 = Increment(x=w1340) -> (x+1=w1339:T7)
      }
      frame "Warn if Current Calibration fit is poor" {
        w1373 = FALSE  # Dialog Box (T)
        n549 = local read "Coefficients"() -> (w1375:dbl[][])
        n550 = local read "Root Name"() -> (w1372:string[])
        n551 = for {
          tunnel: w1375 -> [w1383] mode=indexing
          shift-right: [w1385] -> w1370
          shift-left: "" -> [w1386]
          tunnel: w1372 -> [w1387] mode=indexing
          tunnel: [w1380] -> w1368 mode=indexing
          tunnel: 2.3 ("t") -> [w1379]
          n552 = Index Array(array=w1383, index=0 ("Index")) -> (element=w1381:dbl)
          n553 = Absolute Value(x=w1381) -> (abs(x)=w1380:dbl)
          n554 = Less?(x=w1380, y=w1379) -> (x < y?=w1384:bool)
          n555 = case shown="False" w1384 {
            tunnel: w1387 -> [w1389 _]
            tunnel: w1380 -> [w1390 _]
            tunnel: w1386 -> [w1393 w1394]
            tunnel: [w1391 w1394] -> w1385
            frame False {
              n556 = Format Into String(format string="The calibration for %s has an average fit error of %.1f%%\\n" ("Format String"), w1389, w1390) -> (resulting string=w1392:string)  [unwired: 2 in, 1 out]
              n557 = Concatenate Strings(w1393, w1392) -> (w1391:string)
            }
            frame True {
            }
          }
        }
        n558 = Array Max & Min(array=w1368) -> (max value=w1367:dbl)  [unwired: 3 out]
        n559 = Greater?(x=w1367, y=7.0) -> (0:w1361:bool)
        n560 = case shown="False" w1361 {
          tunnel: ["Poor Calibration" "Very Poor Calibration"] -> w1360
          frame False {
          }
          frame True {
          }
        }
        n561 = Empty String/Path?(string/path=w1370) -> (empty?=w1362:bool)
        n562 = Not(x=w1362) -> (.not. x?=w1363:bool)
        n563 = Bundle By Name(cluster=errorcluster {"status"=FALSE, "code"=0, "source"=""} ("error in (no error)"), "source"=w1370, "status"=w1363) -> (w1369:errorcluster)
        n564 = call "EnFlo_Error_Handler.vi"("error in (no error)"=w1369, "Error Type"=w1360, "Dialog Box (F)"=w1373) -> ()  [unwired: 3 out]
      }
      frame "Warn if Calibration Coefficients have significantly altered" {
        w1421 = FALSE  # Dialog Box (T)
        w1409 = 8.0 ("y")
        n565 = Unbundle By Name(w1401) -> ("Extra Commands"=w1400:string)
        n566 = local read "New Calib Filenames"() -> (w1414:path[])
        n567 = global read "Extra_Commands_Global.vi" "If Command"() -> (w1402:string)
        n568 = global read "Calib_global.vi" "Instrument type"() -> (w1412:T25)
        n569 = local read "Root Name"() -> (w1413:string[])
        n570 = call "Extra_Commands.vi"("String to Search"=w1400, "Command"=w1402) -> ("String Value"=w1399:string)  [unwired: 1 in, 4 out]
        n571 = call "Get_array_values_fr_String.vi"("String Value"=w1399) -> ("Numeric Array"=w1398:dbl[], "String array"=w1404:string[])
        n572 = call "Calibration_Analysis.vi"("Root Name"=w1413, "New Calib Filenames"=w1414, "Instrument type"=w1412, "Clear Calib History"="Clear Calib History") -> ("Error String"=w1411:string, "Max % Error"=w1397:dbl)
        n573 = Index Array(array=w1404, index=0 ("Index")) -> (element=w1405:string)
        n574 = case shown="\"Drift Greater Than\"" w1405 {
          tunnel: w1398 -> [w1429 _]
          tunnel: w1397 -> [w1424 _]
          tunnel: [w1426 w1439] -> w1395
          tunnel: w1396 -> [w1425 w1439]
          frame "Drift Greater Than" {
            n575 = Index Array(array=w1429, index=1 ("Index")) -> (element=w1428:dbl)
            n576 = Greater?(x=w1424, y=w1428) -> (0:w1427:bool)
            n577 = case shown="True" w1427 {
              tunnel: [w1431 w1436] -> w1426
              tunnel: w1425 -> [w1431 w1437]
              tunnel: w1424 -> [_ w1433]
              frame False {
              }
              frame True {
                n578 = Format Into String(format string="Calibration Drift %d%%", w1433) -> (resulting string=w1432:string)  [unwired: 2 in, 1 out]
                n579 = Bundle By Name(cluster=w1437, "Status"=Multi_Run_Status."Jump To Fall Back", "Error Description"=w1432) -> (w1438:T17)
                n580 = call "Merge_Status_Clusters.vi"("Status Cluster 2"=w1438, "Status Cluster 1"=w1437) -> ("Status Cluster Out"=w1436:T17)
              }
            }
          }
          frame "No Match", Default {
          }
        }
        n581 = Format Into String(format string="Calibration Drift Greater than %d%%", w1409) -> (resulting string=w1407:string)  [unwired: 2 in, 1 out]
        n582 = Greater?(x=w1397, y=w1409) -> (0:w1410:bool)
        n583 = Select(t=w1407, s=w1410, f="Calibration Drift") -> (s? t:f=w1415:string)
        n584 = Empty String/Path?(string/path=w1411) -> (empty?=w1419:bool)
        n585 = Not(x=w1419) -> (.not. x?=w1418:bool)
        n586 = Bundle By Name(cluster=errorcluster {"status"=FALSE, "code"=0, "source"=""} ("error in (no error)"), "source"=w1411, "status"=w1418) -> (w1417:errorcluster)
        n587 = call "EnFlo_Error_Handler.vi"("error in (no error)"=w1417, "Error Type"=w1415, "Dialog Box (F)"=w1421) -> ()  [unwired: 3 out]
      }
      frame "Reset Traverse positions" {
        n588 = case shown="\"Concentration\"" w1445 {
          tunnel: w1443 -> [_ w1451]
          tunnel: w1444 -> [_ w1450]
          tunnel: w1442 -> [_ w1449]
          tunnel: w1440 -> [_ w1448]
          frame "Tunnel Speed", Default {
          }
          frame "Concentration" {
            n589 = stacked-sequence {
              tunnel: w1451 -> [_ w1466 _]
              tunnel: w1450 -> [_ w1458 w1474]
              tunnel: w1449 -> [_ w1455 _]
              tunnel: w1448 -> [_ _ w1473]
              frame #0 {
                n590 = global write "Trav_pos_global.vi" "Bkgnd Number Since Calibration"(0 ("Bkgnd Number Since Calibration")) -> ()
              }
              frame #1 {
                n591 = Unbundle By Name(w1466) -> ("Averaging time (mins)"=w1468:dbl)
                n592 = Unbundle By Name(w1466) -> ("Start X"=w1453:sgl, "Start Z"=w1457:sgl)
                n593 = Array Size(array=w1455) -> (size(s)=w1456:i32[])
                n594 = Index Array(array=w1456) -> (element=w1454:i32)  [unwired: 1 in]
                n595 = Multiply(x=60.0, y=w1468) -> (x*y=w1465:dbl)
                n596 = Add(x=w1465, y=60.0) -> (x+y=w1463:dbl)
                n597 = Multiply(x=w1463, y=w1454) -> (x*y=w1462:dbl)
                n598 = global read "Trav_pos_global.vi" "Simulation Time"() -> (w1461:timestamp)
                n599 = Add(x=w1457, y=50.0) -> (x+y=w1469:dbl)
                n600 = Add(x=w1461, y=w1462) -> (x+y=w1459:timestamp)
                n601 = Bundle By Name(cluster=w1466, "Start X"=w1453, "Start Z"=w1469) -> (w1470:T1)
                n602 = call "Set_Traverse_Position.vi"("Currently on Point"=1, "Simulate/Run"=w1458, "Traverse line"=w1470) -> ()  [unwired: 3 in, 1 out]
                n603 = call "Run_FFID_Bkgnd.vi"("Simulated Time"=w1459, "Run Now?"=TRUE, "Simulate/Run"=w1458) -> ()  [unwired: 3 out]
              }
              frame #2 {
                n604 = case shown="\"Run VI\"" w1474 {
                  tunnel: w1473 -> [_ w1475]
                  frame "Check VI only", Default {
                  }
                  frame "Run VI" {
                    n605 = case shown="True" w1475 {
                      frame False {
                      }
                      frame True {
                        n606 = call "ASYNC_Adam_client.vi"("Values"=dbl[] [0.0], "Channel Names"=string[] ["GMU:Mains Divertor:Valve"]) -> ()  [unwired: 1 in, 2 out]
                      }
                    }
                  }
                }
              }
            }
          }
        }
      }
      frame "Post Process Raw Data Files" {
        # "If you want to PP files put this in the Multi run program as a Run Vi Named \"Post Process Files in MultiRun.vi\""
      }
      frame "End" {
        n607 = local write "Clear Calib History"(FALSE ("Clear Calib History")) -> ()
      }
    }
    "Currently in Case" <- w41
  }
  n608 = Unbundle By Name(w12) -> ("Error Description"=→"Error Messages":string, "Status"=→"Status":T6)
